vi "VP_NanoPositioner_FPGA_ModTrans.vi"() -> ()   [LabVIEW 2015]
uses:
  FPGA states.ctl
  FPGA Commands.ctl
  RT VIs/Scan type.ctl
  Data Save Trigger.ctl
  Scan Geometry.ctl
  spiral radial direction.ctl
  spiral rotation direction.ctl
  Inner Scan axis.ctl
  Scan Type and Geometry.ctl
  Data Save Flag.ctl
  <vilib>/Platform/TimedLoop/XDataNode/timing_clust.ctl
  <vilib>/Platform/TimedLoop/XDataNode/nitl_modes.ctl
  <vilib>/Platform/TimedLoop/XDataNode/wakeup.ctl
  Trajectory FGV states.ctl
  Transfer_function_coeffs.ctl
  Transfer_function_actions.ctl
  <vilib>/rvi/Emulation/niFpgaGetClockAttributes.vi
  <vilib>/rvi/Emulation/niFpgaSctlEmulationGetInTimedLoop.vi
  <vilib>/rvi/Emulation/niFpgaEmulationReportErrorSimple.vi
  <vilib>/rvi/Emulation/niFpgaEmulationIsFPGAContextNoSignature.vi
  <vilib>/rvi/DataTransferAndStorage/Container/Common/niFpgaContainerGetUniqueNameForEmu.vi
  <vilib>/rvi/Memory/Memory_Emulation/niFpgaMemoryEmulationCacheClearOnFirstRun.vi
  <vilib>/rvi/Memory/Memory_Emulation/nirvimemoryEmulationManagerCache_MakeExclusive.vi
  <vilib>/rvi/Memory/Memory_Emulation/niFpgaMemoryEmulationValidateCache.vi
  <vilib>/rvi/Memory/Memory_Emulation/nirvimemoryEmulationManagerCache_InsertValue.vi
  <vilib>/Utility/error.llb/Clear Errors.vi
  <vilib>/rvi/Memory/Memory_Emulation/nirvimemoryEmulationManagerCache_ReleaseExclusive.vi
  <vilib>/rvi/Memory/Memory_Emulation/nirvimemoryEmulationManagerCache_GetValue.vi
  <vilib>/rvi/Memory/Memory_Emulation/nirvimemoryEmulationManagerCache_SetValue.vi
  <vilib>/rvi/Emulation/niFpgaProcessEmulError.vi
  <vilib>/rvi/Emulation/niFpgaCriticalErrorInLSC.vi
  <vilib>/rvi/interface/RandomDataEmulation/niFpgaRandomDataHandleErrors.vi
  <vilib>/rvi/eio/common/nirviEmuTemplateMethod_errors.vi
  <vilib>/rvi/DataTransferAndStorage/Container/XNode/niFpgaContainer.xnode
  <vilib>/rvi/DataTransferAndStorage/Register/Emulation/niFpgaRegisterEmulation.vi
  <vilib>/rvi/interface/RandomDataEmulation/nirviRandomDataFpgaReadWriteTemplate.vi
  <vilib>/eio/EIONode/EIONode.xnode
  <vilib>/Platform/TimedLoop/XDataNode/XDataNode.xnode
  <vilib>/Platform/TimedLoop/XDataNode/XDNodeRunTimeDep.lvlib
panel:
  in  "Data Save Flag":T1=enum."Save Data"
  out "Position Number":u32
  out "Scan Type and Geometry":T2
  out "Outer Loop iterations":i32
  out "Counter Loop iterations":i32
  in  "Y Reference DC Offset (nm)":fxp<+/-,16,16>
  in  "Y Reference Amplitude (nm)":fxp<+/-,40,17>
  in  "X Reference DC Offset (nm)":fxp<+/-,16,16>
  in  "X Reference Amplitude (nm)":fxp<+/-,40,17>
  out "Controller loop iterations":i32
  out "Trajectory Complete":bool
  in  "Inner Scan axis":T3
  in  "Spiral Rotation Direction":T4
  in  "Radial direction":T5=enum."Inward"
  in  "Det Frequency":fxp<+,32,0>=0.9999999997671694
  in  "Traj Frequency":fxp<+,32,0>=0.9999999997671694
  in  "Max radius":fxp<+/-,32,16>
  in  "Spiral Step Size":fxp<+/-,32,16>
  in  "Y Step Size":fxp<+/-,24,16>
  in  "X Step Size":fxp<+/-,24,16>
  in  "Scan Geometry":T6
  out "Z Reference Loop iterations":i32
  out "XY Reference Loop iterations":i32
  in  "Data Save Trigger Source":T7
  out "FIFO loop iterations":i32
  out "Trigger Generation Loop iterations":i32
  out "Module output loop iterations":i32
  out "Plant output loop iterations":i32
  in  "Scan type":T8
  out "Interferometer Loop Error":errorcluster
  out "Wait error":errorcluster
  out "Shutdown error":errorcluster
  out "FPGA error monitor":errorcluster
  out "Run Loop error":errorcluster
  in  "Wait timer (ms)":u16=50 caption="Count(mSec)"
  in  "New FPGA command":bool
  in  "FPGA command":T9
  out "FPGA state":T10
  out "End Run Error":errorcluster
  in  "Y End (nm)":fxp<+/-,16,16>
  in  "Y Start (nm)":fxp<+/-,16,16>
  in  "X End (nm)":fxp<+/-,16,16>
  in  "X Start (nm)":fxp<+/-,16,16>
  in  "DT Reset":bool
  in  "DT Duty Cycle (periods)":fxp<+,32,0>=0.5 caption="DT duty cycle (periods)"
  in  "DT Reference DC Offset (V)":fxp<+/-,16,16>
  in  "DT Reference Amplitude (V)":fxp<+/-,40,17>
  in  "DT Phase Offset (periods)":fxp<+,32,0>
  out "Measured Z Reference Loop Period (ticks)":u32
  in  "Z Reference Loop Period (us)":u32 caption="Z Reference Time Period (uSec)"
  in  "Z Reference DC Offset (nm)":fxp<+/-,16,16>
  in  "Z Reference Amplitude (nm)":fxp<+/-,40,17>
  in  "Detector Trigger Lower Limit (V)":fxp<+/-,20,5>=-5.0
  out "Detector Trigger In Range?":bool
  in  "Detector Trigger Upper Limit (V)":fxp<+/-,20,5>=5.0
  out "Measured Trigger Generation Loop Period (Ticks)":u32
  in  "Trigger Generation Time Period (uSec)":u32
  in  "Z-Stage Scaling Direction":fxp<+/-,3,3>=-1.0
  in  "Y-Stage Scaling Direction":fxp<+/-,3,3>=-1.0
  in  "Optics and or Sample Stage":T11(ring)
  in  "Sample Z Stage Resolution (nm)":fxp<+,33,3>=0.001000046730041504
  in  "Sample Y Stage Resolution (nm)":fxp<+,33,3>=0.001000046730041504
  in  "Sample X Stage Resolution (nm)":fxp<+,33,3>=0.001000046730041504
  out "Sample Z Stage Displacement raw (nm)":fxp<+/-,32,16> format="%.62g"
  out "Sample Y Stage Displacement raw (nm)":fxp<+/-,32,16> format="%.41g"
  out "Sample X Stage Displacement raw (nm)":fxp<+/-,32,16> format="%.62g"
  in  "Reset Sample Z":bool
  in  "Reset Sample Y":bool
  in  "Reset Sample X":bool
  out "Mod6/DIO3":bool
  out "Mod6/DIO2":bool
  out "Mod5/DIO3":bool
  out "Mod5/DIO2":bool
  out "Mod4/DIO3":bool
  out "Mod4/DIO2":bool
  in  "X-Stage Scaling Direction":fxp<+/-,3,3>=-1.0
  in  "Z-Stage nm to V Scaling":fxp<+/-,32,12>
  in  "Y-Stage nm to V Scaling":fxp<+/-,32,12>
  in  "X-Stage nm to V Scaling":fxp<+/-,32,12>
  out "Kxx Output, Kxx*ex (V)":fxp<+/-,58,25>
  out "Kyy Output, Kyy*ey (V)":fxp<+/-,58,25>
  out "Kzz Output, Kzz*ez (V)":fxp<+/-,58,25>
  in  "sos gain SF Controller xx1":fxp<+/-,42,9>
  in  "-a01(2) xx1":fxp<+/-,64,9>[](array[numeric])=[0.0, 0.0, 0.0, 0.0, 0.0, 0.0, 0.0, 0.0, 0.0, 0.0, 0.0, 0.0, 0.0, 0.0, 0.0, 0.0, 0.0, 0.0, 0.0, 0.0]
  in  "-a02(2) xx1":fxp<+/-,64,9>[](array[numeric])=[0.0, 0.0, 0.0, 0.0, 0.0, 0.0, 0.0, 0.0, 0.0, 0.0, 0.0, 0.0, 0.0, 0.0, 0.0, 0.0, 0.0, 0.0, 0.0, 0.0]
  in  "b01(2) xx1":fxp<+/-,64,9>[](array[numeric])=[0.0, 0.0, 0.0, 0.0, 0.0, 0.0, 0.0, 0.0, 0.0, 0.0, 0.0, 0.0, 0.0, 0.0, 0.0, 0.0, 0.0, 0.0, 0.0, 0.0]
  in  "b02(2) xx1":fxp<+/-,64,9>[](array[numeric])=[0.0, 0.0, 0.0, 0.0, 0.0, 0.0, 0.0, 0.0, 0.0, 0.0, 0.0, 0.0, 0.0, 0.0, 0.0, 0.0, 0.0, 0.0, 0.0, 0.0]
  in  "sos gain SF Controller yy1":fxp<+/-,42,9>
  in  "-a01(2) yy1":fxp<+/-,64,9>[](array[numeric])=[0.0, 0.0, 0.0, 0.0, 0.0, 0.0, 0.0, 0.0, 0.0, 0.0, 0.0, 0.0, 0.0, 0.0, 0.0, 0.0, 0.0, 0.0, 0.0, 0.0]
  in  "-a02(2) yy1":fxp<+/-,64,9>[](array[numeric])=[0.0, 0.0, 0.0, 0.0, 0.0, 0.0, 0.0, 0.0, 0.0, 0.0, 0.0, 0.0, 0.0, 0.0, 0.0, 0.0, 0.0, 0.0, 0.0, 0.0]
  in  "b01(2) yy1":fxp<+/-,64,9>[](array[numeric])=[0.0, 0.0, 0.0, 0.0, 0.0, 0.0, 0.0, 0.0, 0.0, 0.0, 0.0, 0.0, 0.0, 0.0, 0.0, 0.0, 0.0, 0.0, 0.0, 0.0]
  in  "b02(2) yy1":fxp<+/-,64,9>[](array[numeric])=[0.0, 0.0, 0.0, 0.0, 0.0, 0.0, 0.0, 0.0, 0.0, 0.0, 0.0, 0.0, 0.0, 0.0, 0.0, 0.0, 0.0, 0.0, 0.0, 0.0]
  in  "sos gain SF Controller zz1":fxp<+/-,42,9>
  in  "-a01(2) zz1":fxp<+/-,64,9>[](array[numeric])=[0.0, 0.0, 0.0, 0.0, 0.0, 0.0, 0.0, 0.0, 0.0, 0.0, 0.0, 0.0, 0.0, 0.0, 0.0, 0.0, 0.0, 0.0, 0.0, 0.0]
  in  "-a02(2) zz1":fxp<+/-,64,9>[](array[numeric])=[0.0, 0.0, 0.0, 0.0, 0.0, 0.0, 0.0, 0.0, 0.0, 0.0, 0.0, 0.0, 0.0, 0.0, 0.0, 0.0, 0.0, 0.0, 0.0, 0.0]
  in  "b01(2) zz1":fxp<+/-,64,9>[](array[numeric])=[0.0, 0.0, 0.0, 0.0, 0.0, 0.0, 0.0, 0.0, 0.0, 0.0, 0.0, 0.0, 0.0, 0.0, 0.0, 0.0, 0.0, 0.0, 0.0, 0.0]
  in  "b02(2) zz1":fxp<+/-,64,9>[](array[numeric])=[0.0, 0.0, 0.0, 0.0, 0.0, 0.0, 0.0, 0.0, 0.0, 0.0, 0.0, 0.0, 0.0, 0.0, 0.0, 0.0, 0.0, 0.0, 0.0, 0.0]
  in  "Scaling mV to V":fxp<+,33,10>=0.0009765625
  in  "System Loop Type":enum16{"Open Loop", "Closed Loop"}(ring)
  in  "Timeout FPGA FIFO1":i32=40000000
  out "FIFO Timed Out":bool
  out "Number of Data Strings":i32
  out "Optics Z Stage Displacement raw (nm)":fxp<+/-,32,16>
  in  "Optics Z Stage Resolution (nm)":fxp<+,33,3>=0.001000046730041504
  in  "Reset Optics Z":bool
  out "Mod6/DIO1":bool
  out "Mod6/DIO0":bool
  out "Optics Y Stage Displacement raw (nm)":fxp<+/-,32,16>
  in  "Optics Y Stage Resolution (nm)":fxp<+,33,3>=0.001000046730041504
  in  "Reset Optics Y":bool
  out "Mod5/DIO1":bool
  out "Mod5/DIO0":bool
  out "Z-Stage Input In Range?":bool
  out "Y-Stage Input In Range?":bool
  in  "Controller Output Lower Limit":fxp<+/-,20,5>=-5.0
  out "X-Stage Input In Range?":bool
  in  "Controller Output Upper Limit":fxp<+/-,20,5>=5.0
  out "Measured Counter Time Period (Ticks)":u32
  out "Measured Datalog Period (Ticks)":u32
  out "Measured Plant Output Loop Period (Ticks)":u32
  out "Measured Module Output Loop Period (Ticks)":u32
  out "Measured Controller Loop Period (Ticks)":u32
  out "Measured XY Reference Loop Period (ticks)":u32
  out "Optics X Stage Displacement raw (nm)":fxp<+/-,32,16>
  in  "Optics X Stage Resolution (nm)":fxp<+,33,3>=0.001000046730041504 format="%#_31g"
  in  "Plant Output Loop Period (uSec)":u32 caption="Plant Output Time Period (uSec)"
  in  "Reset Optics X":bool
  out "Mod4/DIO1":bool
  out "Mod4/DIO0":bool
  out "Start Run Error":errorcluster
  out "Stop Scan":bool
  in  "Module Output Loop Period (uSec)":u32 caption="Controller Output Time Period (uSec)"
  in  "Datalog Cases":T12(ring)
  in  "Controller Loop Period (uSec)":u32 caption="Controller Time Period (uSec)"
  in  "FIFO Loop Period (us)":u32 caption="Datalog Time Period (uSec)"
  in  "XY Reference Loop Period (us)":u32 caption="X Reference Time Period (uSec)"
  out "FIFO Timed Out?":bool
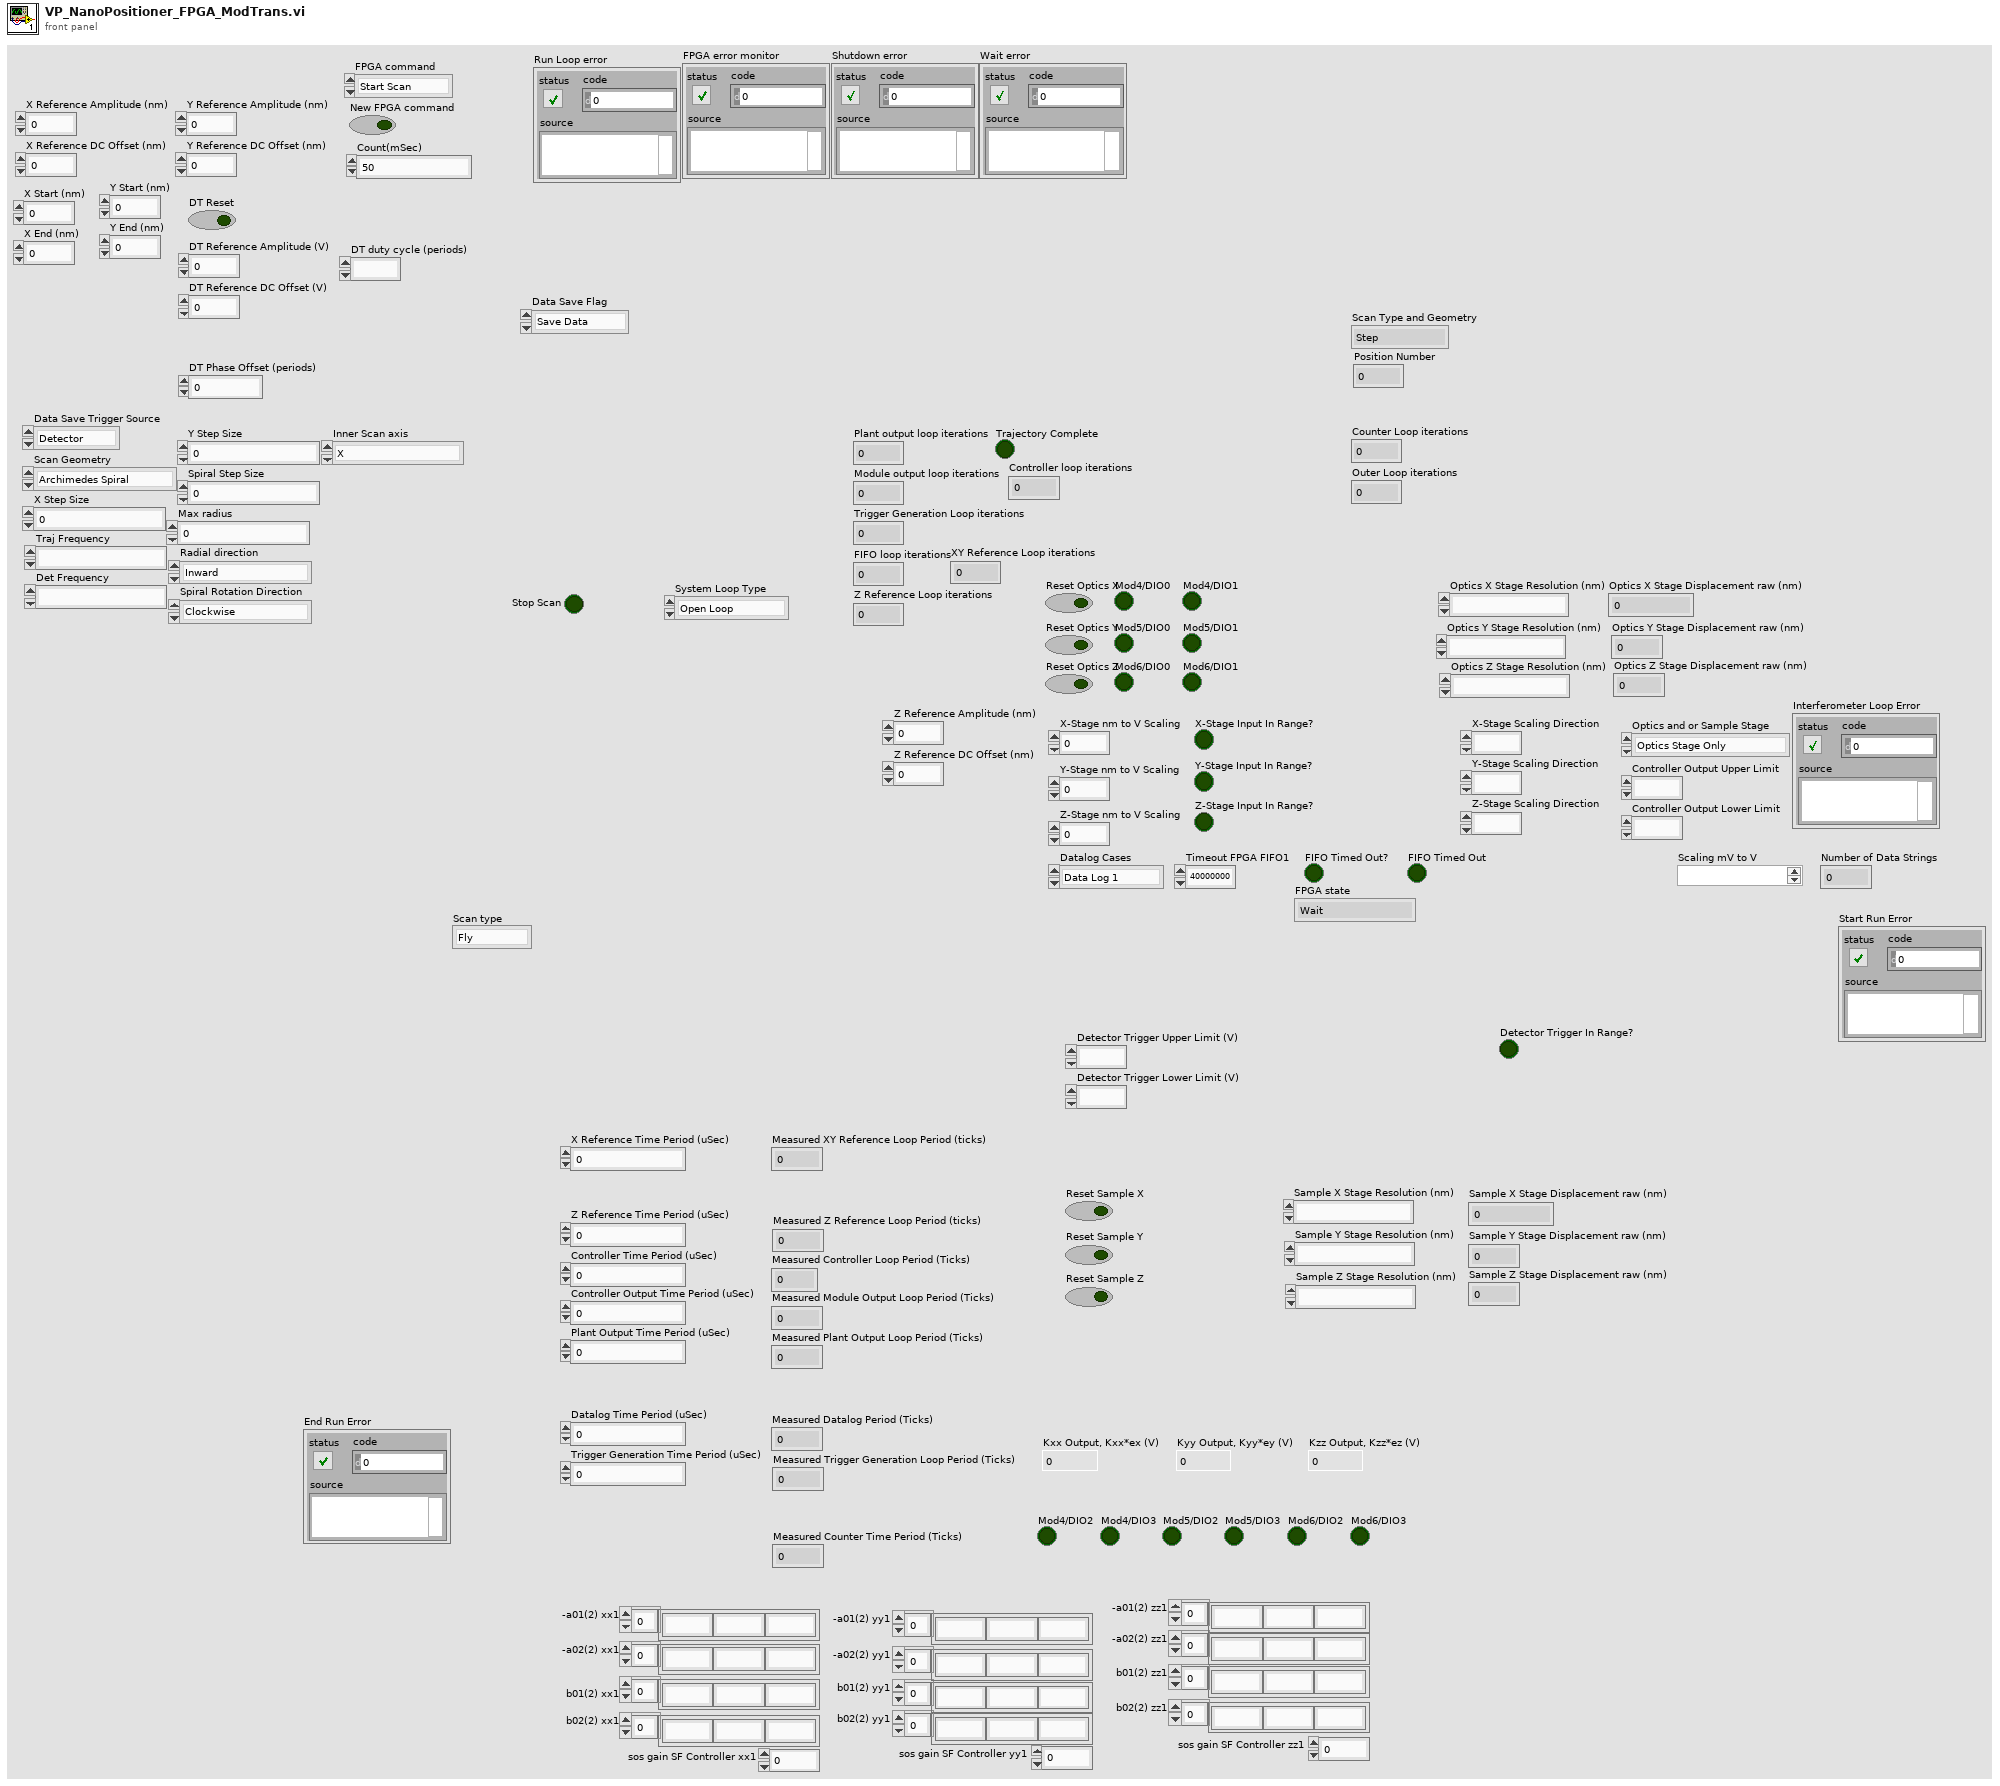
[diagram p1: front panel]
types:
  T1 = typedef "Data Save Flag.ctl" = enum16{"Skip Data", "Save Data"}
  T2 = typedef "Scan Type and Geometry.ctl" = enum16{"Step", "Fly Arch Spiral", "Fly Snake", "Fly Grid Spiral"}
  T3 = typedef "Inner Scan axis.ctl" = enum16{"X", "Y"}
  T4 = typedef "spiral rotation direction.ctl" = enum16{"Clockwise", "Anti-clockwise"}
  T5 = typedef "spiral radial direction.ctl" = enum16{"Outward", "Inward"}
  T6 = typedef "Scan Geometry.ctl" = enum16{"Archimedes Spiral", "Grid Spiral", "Snake"}
  T7 = typedef "Data Save Trigger.ctl" = enum16{"Detector", "Trajectory"}
  T8 = typedef "Scan type.ctl" = enum16{"Fly", "Step"}
  T9 = typedef "FPGA Commands.ctl" = enum16{"Start Scan", "Shutdown"}
  T10 = typedef "FPGA states.ctl" = enum16{"Wait", "Start Run", "Run", "End Run", "Shutdown"}
  T11 = enum16{"Optics Stage Only", "Optics and Sample Stage"}
  T12 = enum16{"Data Log 1", "Data Log 2", "Data Log 3", "Data Log 4", "Data Log 5", "Data Log 6", "Data Log 7", "Data Log 8", "Data Log 9", "Data Log 10", "Data Log 11", "Data Log 12", "Data Log 13", "Data Log 14", "Data Log 15", "Data Log 16"}
  T13 = typedef "Transfer_function_actions.ctl" = enum16{"Initialize", "Calculate"}
  T14 = typedef "Trajectory FGV states.ctl" = enum16{"Initialize", "Increment"}
  T15 = typedef "XDNodeRunTimeDep.lvlib/timing_clust.ctl" = cluster{"Expected End [f-1]":u64, "Actual End [f-1]":u64, "Finished Late? [f-1]":bool, "Expected End [i-1]":u64, "Actual End [i-1]":u64, "Finished Late? [i-1]":bool, "Expected Start [i]":u64, "Actual Start [i]":u64, "Expected Start [f]":u64, "Actual Start [f]":u64, "Source Name":string, "Structure Name":string, "Period":i64, "Deadline":i64, "Offset":i64, "Start":i64, "Priority":i32, "Timeout":i32, "Mode":T16, "Wakeup Reason":T17, "Error":errorcluster, "Source Type":string, "Secondary Source Type":string, "Global End Time":u64, "Global Start Time":u64, "Frame Duration":u64, "Iteration Duration":u64, "Assigned CPU":i32, "I/O Scan Engine Mode":u32}
  T16 = typedef "XDNodeRunTimeDep.lvlib/nitl_modes.ctl" = enum32{"No Change", "Process missed periods, maintain original phase", "Discard missed periods, maintain original phase", "Process missed periods, ignore original phase", "Discard missed periods, ignore original phase"}
  T17 = typedef "XDNodeRunTimeDep.lvlib/wakeup.ctl" = enum32{"Normal", "Aborted", "Asynchronous wakeup", "Timing source error", "Timed loop error", "Timeout"}
  T18 = typedef "Transfer_function_coeffs.ctl" = cluster{"sos gain SF Controller":fxp<+/-,42,9>, "-a01(2)":fxp<+/-,64,9>[], "-a02(2)":fxp<+/-,64,9>[], "b01(2)":fxp<+/-,64,9>[], "b02(2)":fxp<+/-,64,9>[]}
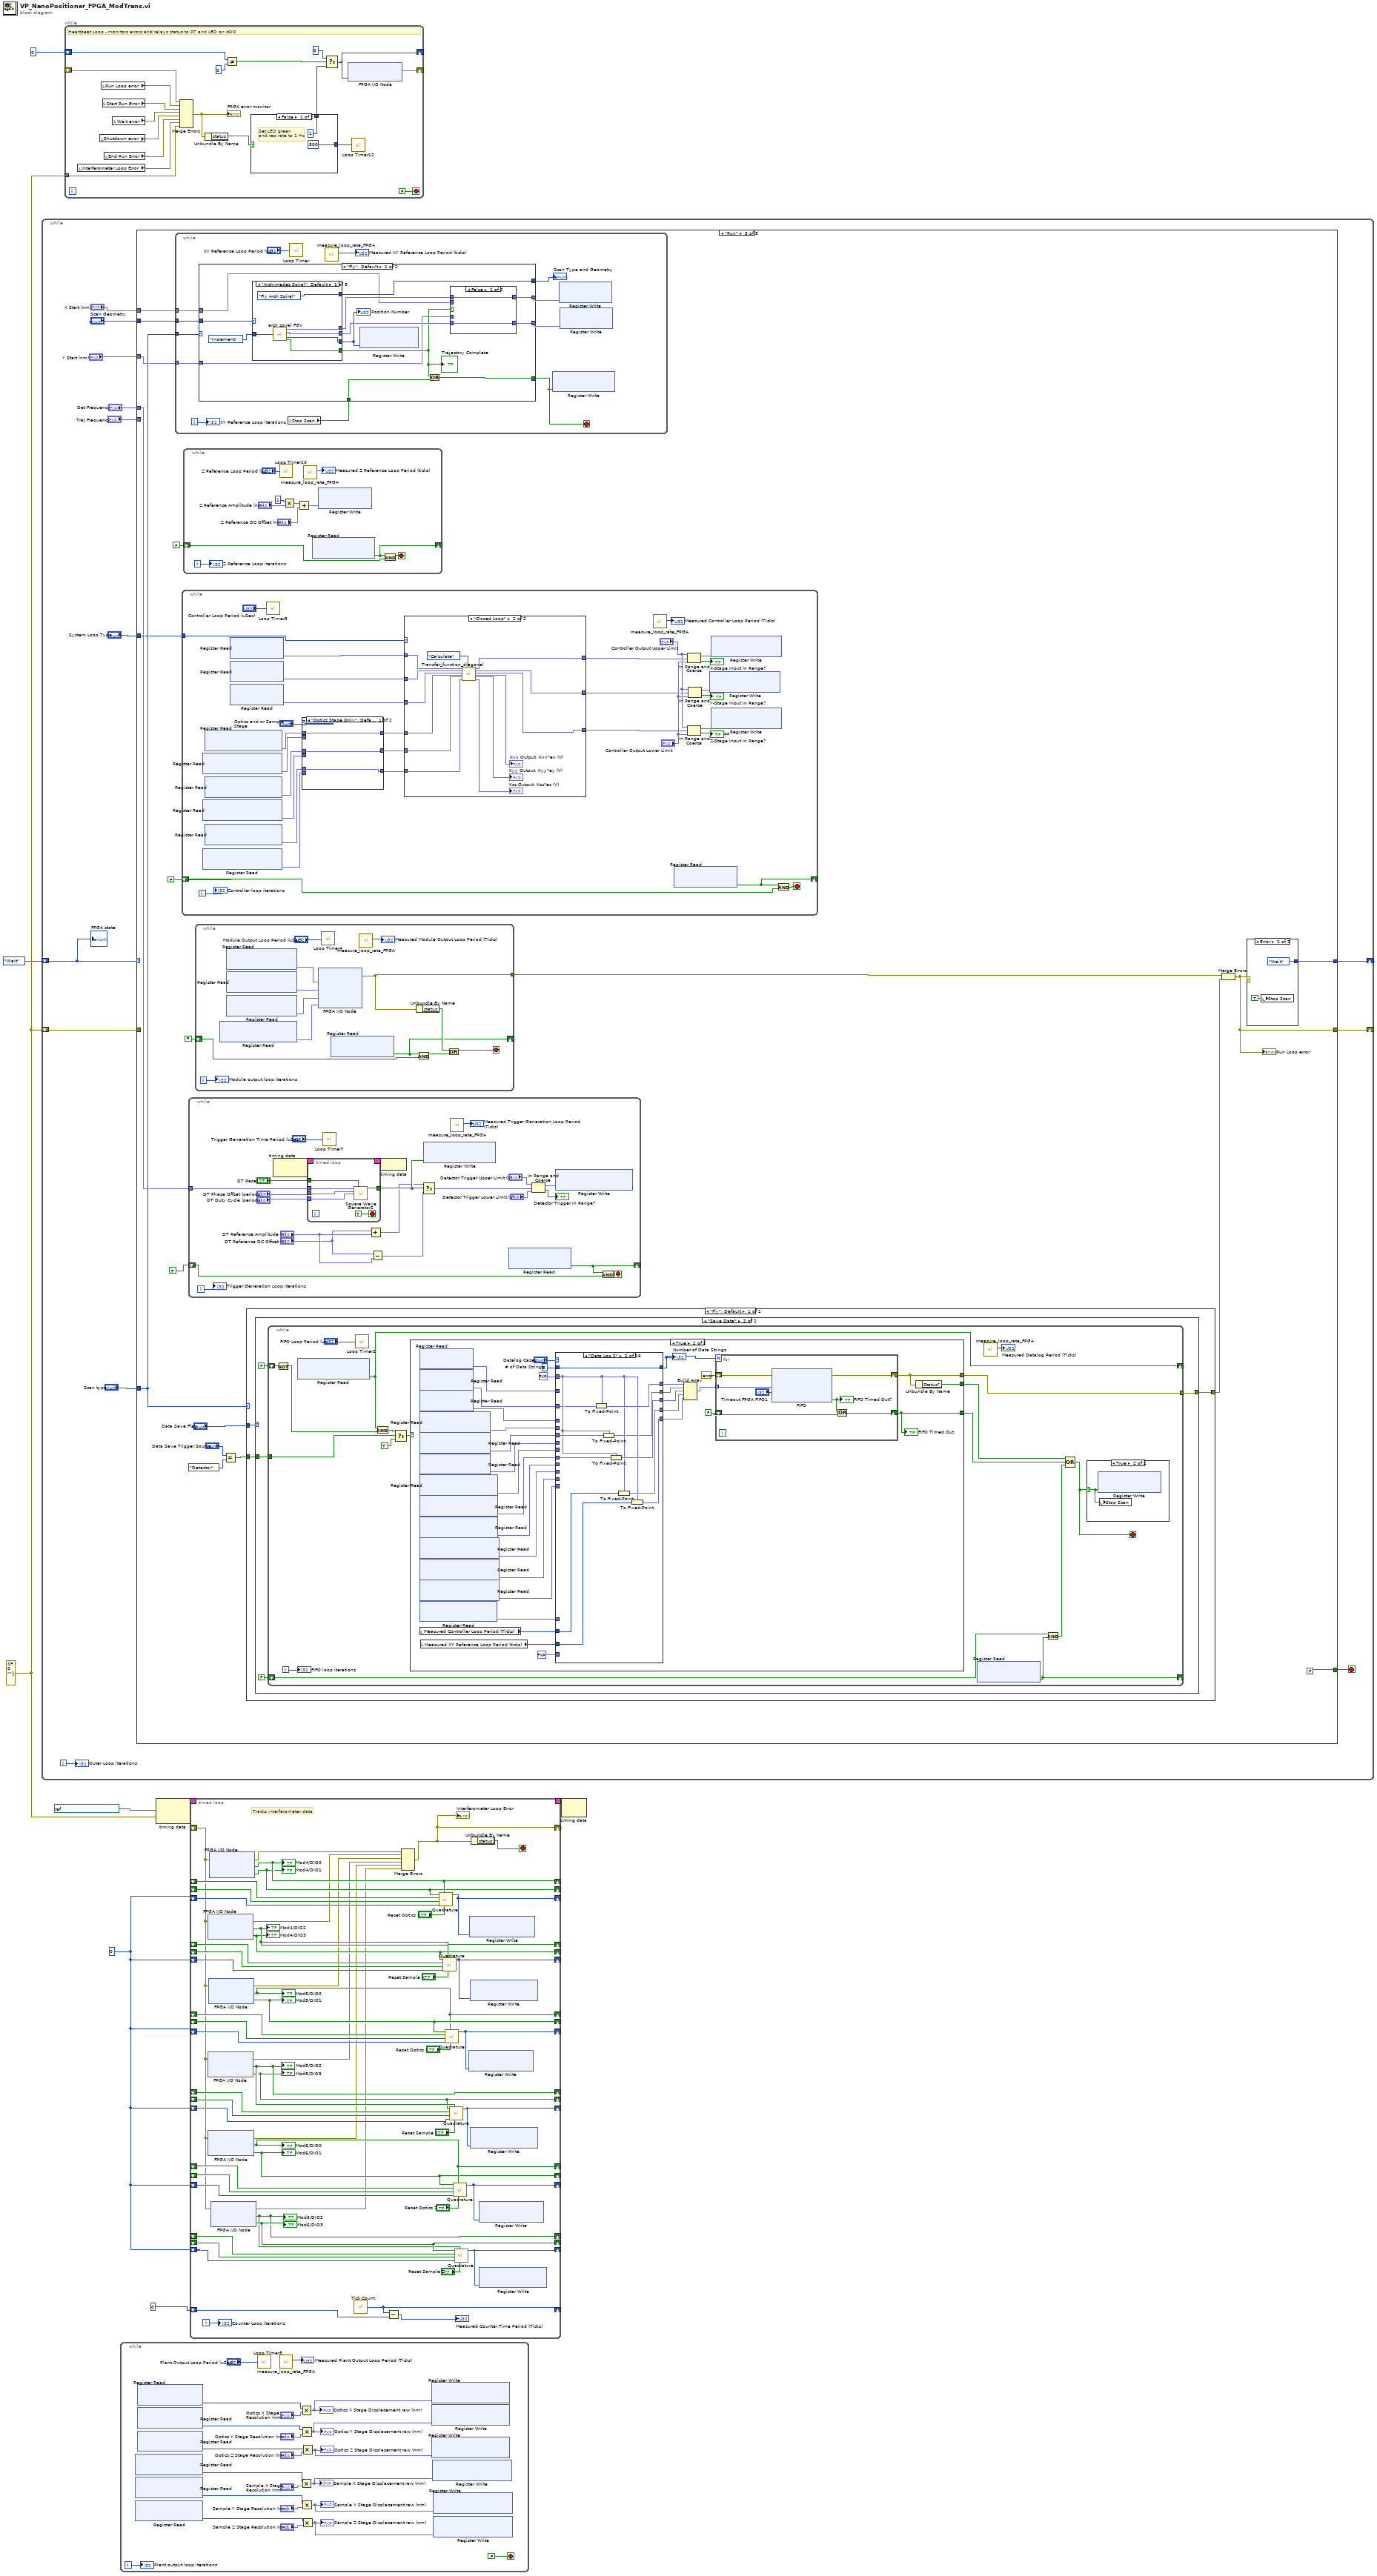
[diagram p0: block diagram]
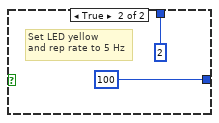
[diagram p2: hidden frame]
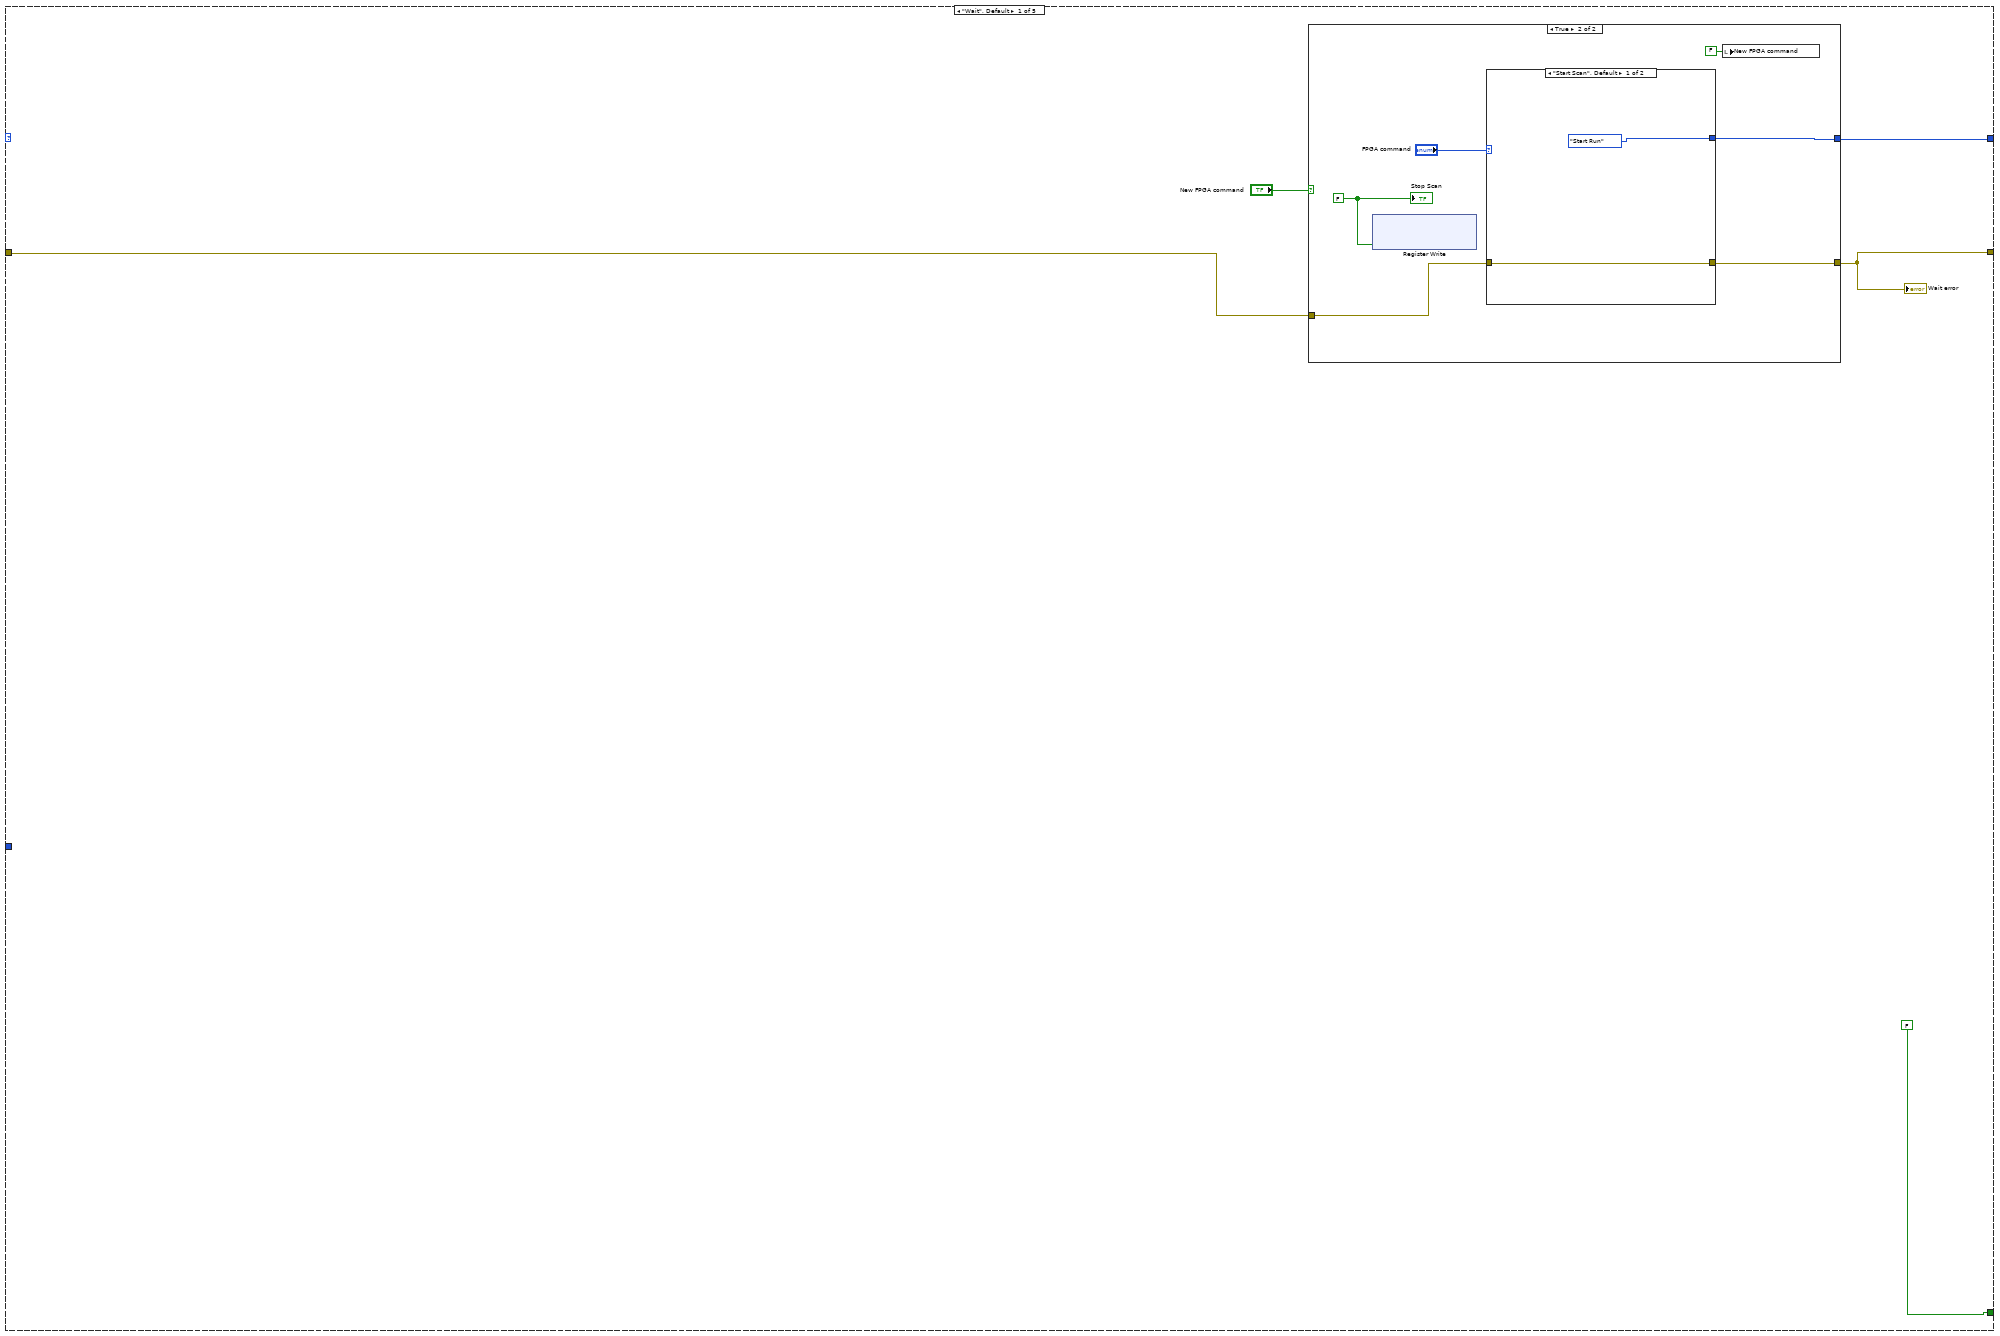
[diagram p3: hidden frame]
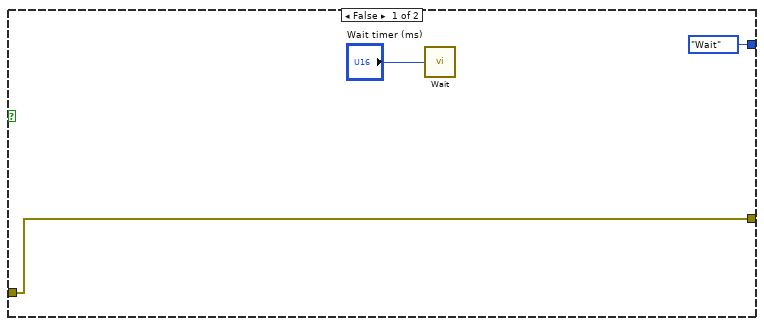
[diagram p4: hidden frame]
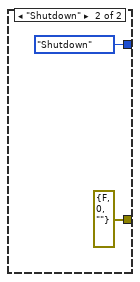
[diagram p5: hidden frame]
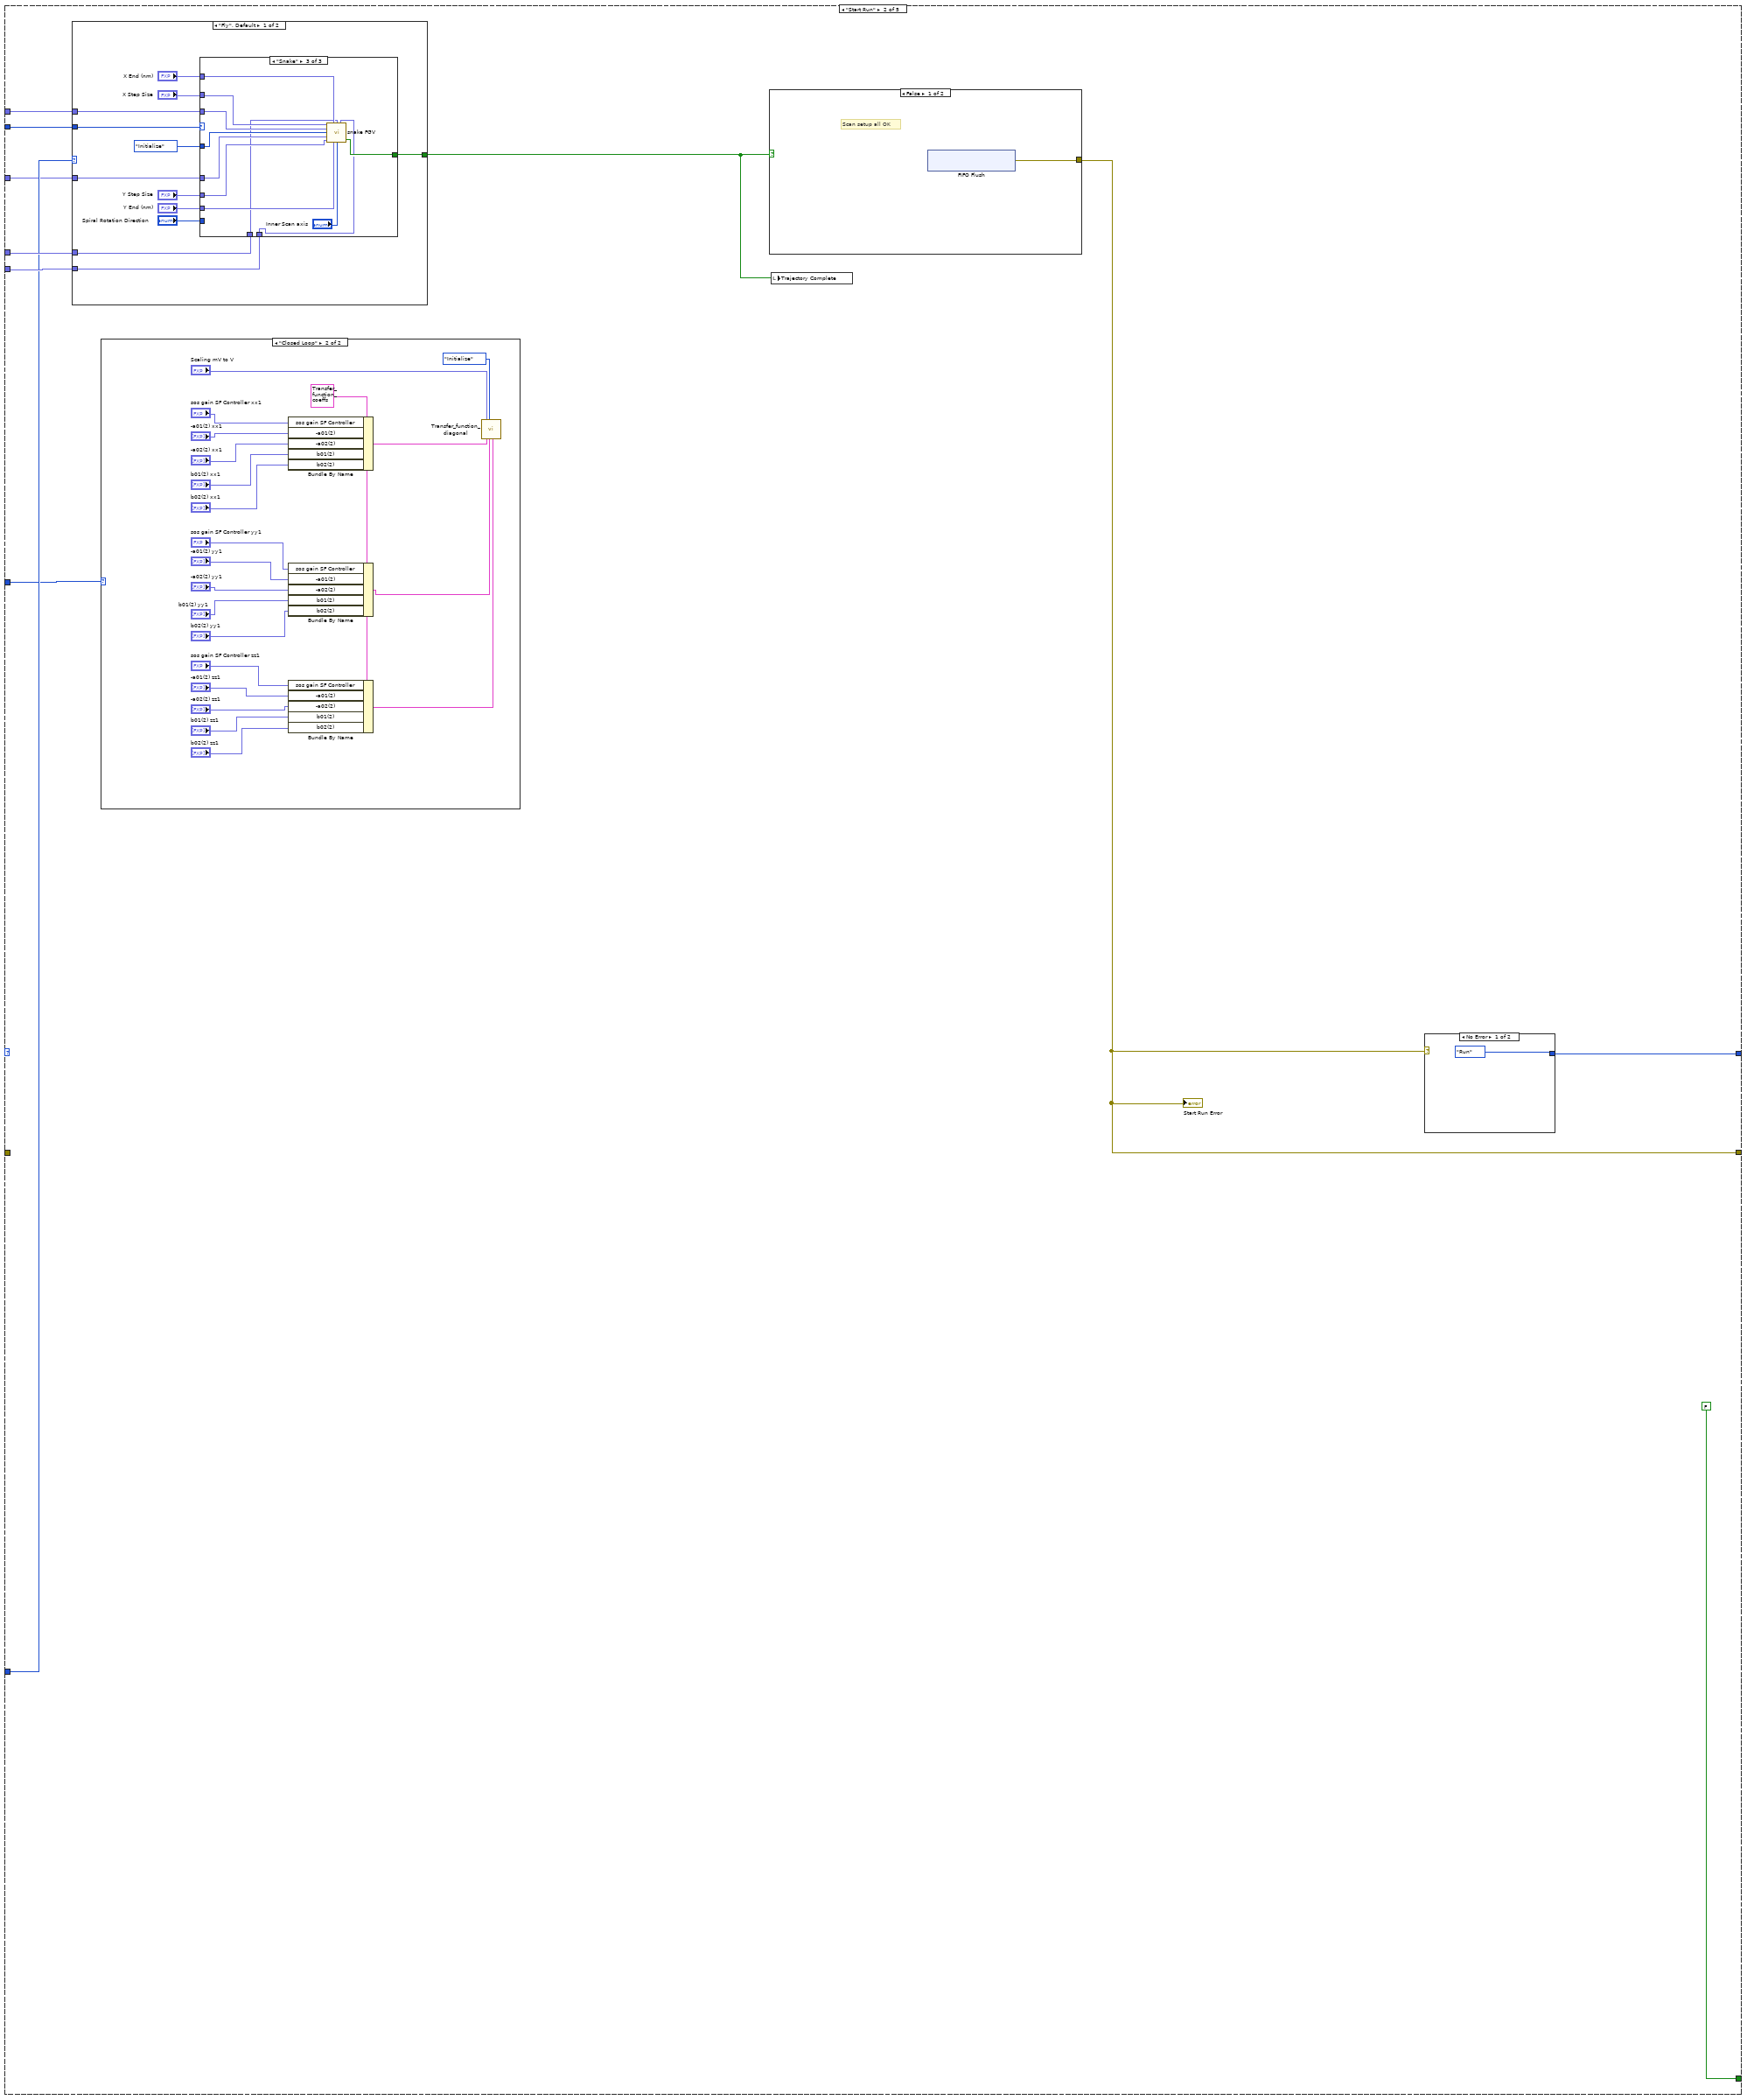
[diagram p6: hidden frame]
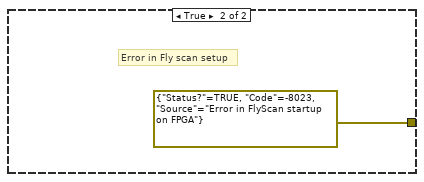
[diagram p8: hidden frame]
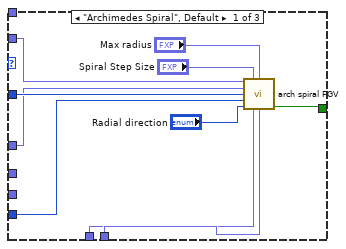
[diagram p9: hidden frame]
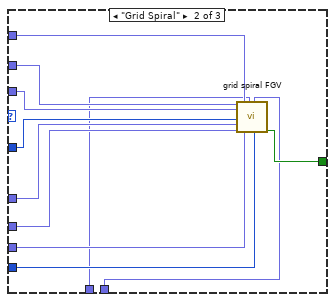
[diagram p10: hidden frame]
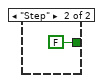
[diagram p11: hidden frame]
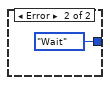
[diagram p12: hidden frame]
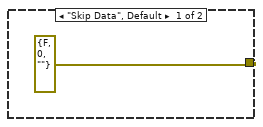
[diagram p13: hidden frame]
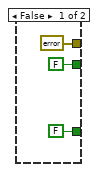
[diagram p14: hidden frame]
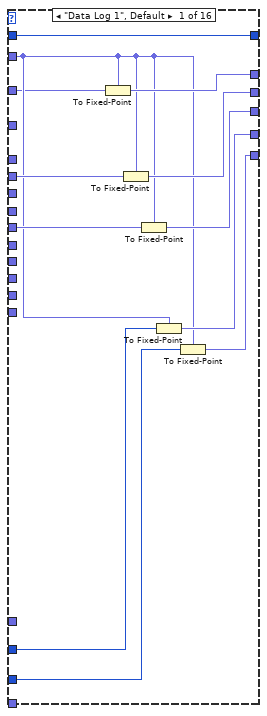
[diagram p15: hidden frame]
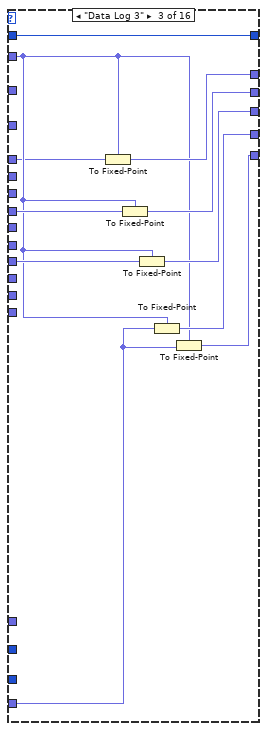
[diagram p16: hidden frame]
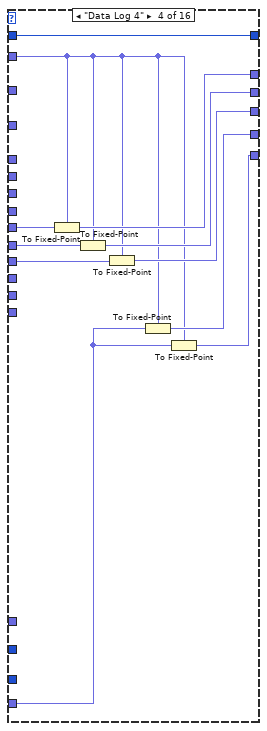
[diagram p17: hidden frame]
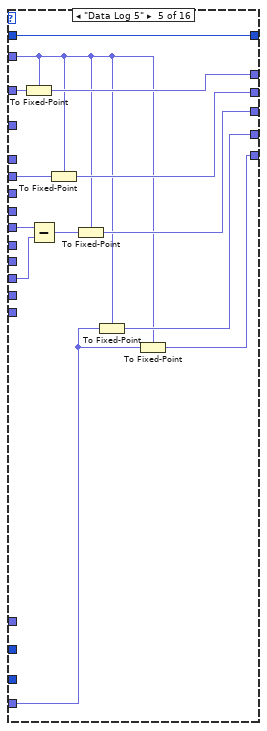
[diagram p18: hidden frame]
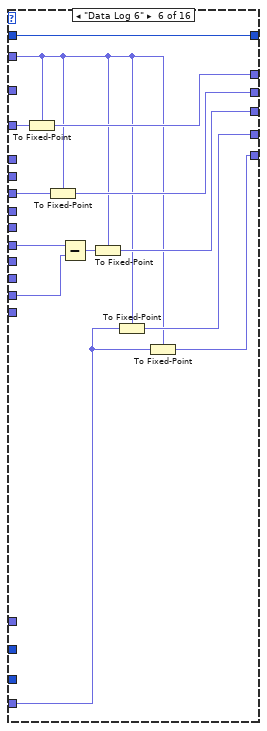
[diagram p19: hidden frame]
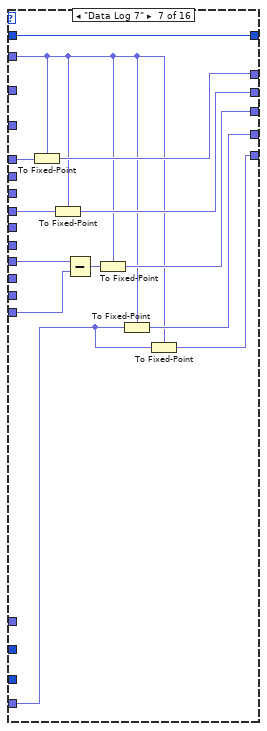
[diagram p20: hidden frame]
diagram:
  w4 = 0 ("Tick Count(Ticks)")
  w1 = errorcluster {"status"=FALSE, "code"=0, "source"=""} ("error IO")
  n1 = while {
    shift-right: [w14] -> _
    shift-left: FPGA_states."Wait" -> [w21]
    shift-right: [w19] -> _
    shift-left: w1 -> [w10]
    i -> [w13]
    stop <- w20 stop-if-true
    n2 = case shown="\"Run\"" w21 {
      tunnel: [w26 w44 w137 w584 w591] -> w19
      tunnel: [FALSE FALSE FALSE FALSE TRUE] -> w20
      tunnel: [w23 w45 w138 FPGA_states."Wait" FPGA_states."Shutdown"] -> w14
      tunnel: w10 -> [w24 _ _ w585 w592]
      tunnel: "Scan Geometry" -> [_ w49 w134 _ _]
      tunnel: "Traj Frequency" -> [_ w48 _ _ _]
      tunnel: "Det Frequency" -> [_ w47 w129 _ _]
      tunnel: "Scan type" -> [_ w46 w130 _ _]
      tunnel: "X Start (nm)" -> [_ w42 w124 _ _]
      tunnel: "Y Start (nm)" -> [_ w41 w125 _ _]
      tunnel: "System Loop Type" -> [_ w40 w121 _ _]
      frame "Wait", Default {
        n3 = case shown="True" "New FPGA command" {
          tunnel: [FPGA_states."Wait" w35] -> w23
          tunnel: w24 -> [w29 w34]
          tunnel: [w29 w33] -> w26
          frame False {
            n4 = call "Wait"("Count(mSec)"="Wait timer (ms)") -> ()  [unwired: 1 out]
          }
          frame True {
            w30 = FALSE ("stop case")
            n5 = xnode ("Register Write")("Data"=w30) -> ()  [unwired: 1 in, 1 out]
            n6 = case shown="\"Start Scan\", Default" "FPGA command" {
              tunnel: [FPGA_states."Start Run" FPGA_states."Shutdown"] -> w35
              tunnel: w34 -> [w36 _]
              tunnel: [w36 errorcluster {"status"=FALSE, "code"=0, "source"=""} ("error IO")] -> w33
              frame "Start Scan", Default {
              }
              frame "Shutdown" {
              }
            }
            n7 = local write "New FPGA command"(FALSE ("New FPGA command")) -> ()
            "Stop Scan" <- w30
          }
        }
        "Wait error" <- w26
      }
      frame "Start Run" {
        n8 = case shown="\"Fly\", Default" w46 {
          tunnel: w49 -> [w84 _]
          tunnel: w48 -> [w83 _]
          tunnel: w47 -> [w82 _]
          tunnel: [w76 FALSE ("Trajectory Complete")] -> w43
          tunnel: w42 -> [w75 _]
          tunnel: w41 -> [w74 _]
          frame "Fly", Default {
            n9 = case shown="\"Snake\"" w84 {
              tunnel: Trajectory_FGV_states."Initialize" ("Action") -> [w95 w106 w117]
              tunnel: [w94 w105 w116] -> w76
              tunnel: w75 -> [w93 w104 w115]
              tunnel: "X Step Size" -> [_ w103 w114]
              tunnel: "X End (nm)" -> [_ w102 w113]
              tunnel: w74 -> [w92 w101 w112]
              tunnel: "Y Step Size" -> [_ w100 w111]
              tunnel: "Y End (nm)" -> [_ w99 w110]
              tunnel: w83 -> [w89 w96 w108]
              tunnel: w82 -> [w88 w97 w109]
              tunnel: "Spiral Rotation Direction" -> [w86 w98 _]
              frame "Archimedes Spiral", Default {
                n10 = call "arch spiral FGV.vi"("X Start"=w93, "Spiral Step Size"="Spiral Step Size", "Max radius"="Max radius", "Y Start"=w92, "Action"=w95, "Spiral Rotation Direction"=w86, "Radial direction"="Radial direction", "Det Frequency"=w88, "Traj Frequency"=w89) -> ("Trajectory Complete"=w94:bool)  [unwired: 3 in, 3 out]
              }
              frame "Grid Spiral" {
                n11 = call "grid spiral FGV.vi"("X Step Size"=w103, "X Start"=w104, "Action"=w106, "Y Start"=w101, "Y Step Size"=w100, "X End"=w102, "Y End"=w99, "Det Frequency"=w97, "Traj Frequency"=w96, "Spiral Rotation Direction"=w98) -> ("Trajectory Complete"=w105:bool)  [unwired: 2 in, 7 out]
              }
              frame "Snake" {
                n12 = call "snake FGV.vi"("X Step Size"=w114, "X End"=w113, "Det Frequency"=w109, "Traj Frequency"=w108, "X Start"=w115, "Action"=w117, "Y Start"=w112, "Y Step Size"=w111, "Y End"=w110, "Inner Scan axis"="Inner Scan axis") -> ("Trajectory Complete"=w116:bool)  [unwired: 2 in, 3 out]
              }
            }
          }
          frame "Step" {
          }
        }
        n13 = case shown="\"Closed Loop\"" w40 {
          frame "Open Loop", Default {
          }
          frame "Closed Loop" {
            w71 = T18 {"sos gain SF Controller"=0.0, "-a01(2)"=[0.0, 0.0, 0.0, 0.0, 0.0, 0.0, 0.0, 0.0, 0.0, 0.0, 0.0, 0.0, 0.0, 0.0, 0.0, 0.0, 0.0, 0.0, 0.0, 0.0], "-a02(2)"=[0.0, 0.0, 0.0, 0.0, 0.0, 0.0, 0.0, 0.0, 0.0, 0.0, 0.0, 0.0, 0.0, 0.0, 0.0, 0.0, 0.0, 0.0, 0.0, 0.0], "b01(2)"=[0.0, 0.0, 0.0, 0.0, 0.0, 0.0, 0.0, 0.0, 0.0, 0.0, 0.0, 0.0, 0.0, 0.0, 0.0, 0.0, 0.0, 0.0, 0.0, 0.0], "b02(2)"=[0.0, 0.0, 0.0, 0.0, 0.0, 0.0, 0.0, 0.0, 0.0, 0.0, 0.0, 0.0, 0.0, 0.0, 0.0, 0.0, 0.0, 0.0, 0.0, 0.0]} ("Transfer Function coeffs")
            n14 = Bundle By Name(cluster=w71, "sos gain SF Controller"="sos gain SF Controller xx1", "-a01(2)"="-a01(2) xx1", "-a02(2)"="-a02(2) xx1", "b01(2)"="b01(2) xx1", "b02(2)"="b02(2) xx1") -> (w53:T18)
            n15 = Bundle By Name(cluster=w71, "sos gain SF Controller"="sos gain SF Controller yy1", "-a01(2)"="-a01(2) yy1", "-a02(2)"="-a02(2) yy1", "b01(2)"="b01(2) yy1", "b02(2)"="b02(2) yy1") -> (w52:T18)
            n16 = Bundle By Name(cluster=w71, "sos gain SF Controller"="sos gain SF Controller zz1", "-a01(2)"="-a01(2) zz1", "-a02(2)"="-a02(2) zz1", "b01(2)"="b01(2) zz1", "b02(2)"="b02(2) zz1") -> (w51:T18)
            n17 = call "Transfer_function_diagonal.vi"("Scaling mV to V"="Scaling mV to V", "xx1 Transfer Function"=w53, "Action"=Transfer_function_actions."Initialize", "yy1 Transfer Function"=w52, "zz1 Transfer Function"=w51) -> ()  [unwired: 9 in, 6 out]
          }
        }
        n18 = case shown="False" w43 {
          tunnel: [w72 errorcluster {"Status?"=TRUE, "Code"=-8023, "Source"="Error in FlyScan startup on FPGA"} ("error out")] -> w44
          frame False {
            # "Scan setup all OK"
            n19 = xnode ("FIFO Flush")() -> ("error out"=w72:errorcluster)  [unwired: 2 in, 1 out]
          }
          frame True {
            # "Error in Fly scan setup"
          }
        }
        "Start Run Error" <- w44
        n20 = local write "Trajectory Complete"(w43) -> ()
        n21 = case shown="No Error" w44 {
          tunnel: [FPGA_states."Run" FPGA_states."Wait"] -> w45
          frame No Error {
          }
          frame Error {
          }
        }
      }
      frame "Run" {
        n22 = while {
          tunnel: w134 -> [w537]
          tunnel: w130 -> [w532]
          tunnel: w125 -> [w530]
          tunnel: w124 -> [w529]
          i -> [w538]
          stop <- w533 stop-if-true
          n23 = local read "Stop Scan"() -> (w534:bool)
          n24 = case shown="\"Fly\", Default" w532 {
            tunnel: w537 -> [w553 _]
            tunnel: [w546 w580] -> w536
            tunnel: [w544 w577] -> w535
            tunnel: w534 -> [w550 w583]
            tunnel: [w549 w583] -> w533
            tunnel: [w548 Scan_Type_and_Geometry."Step"] -> w531
            tunnel: w530 -> [w542 _]
            tunnel: w529 -> [w541 _]
            frame "Fly", Default {
              n25 = case shown="\"Archimedes Spiral\", Default" w553 {
                tunnel: Trajectory_FGV_states."Increment" ("Action") -> [w563 w569 w575]
                tunnel: [w562 w568 w574] -> w543
                tunnel: [w561 w567 w573] -> w547
                tunnel: [w560 w566 w572] -> w545
                tunnel: [w559 w565 w571] -> w551
                tunnel: [Scan_Type_and_Geometry."Fly Arch Spiral" Scan_Type_and_Geometry."Fly Grid Spiral" Scan_Type_and_Geometry."Fly Snake"] -> w548
                frame "Archimedes Spiral", Default {
                  n26 = call "arch spiral FGV.vi"("Action"=w563) -> ("X position"=w561:fxp<+/-,32,16>, "Y position"=w560:fxp<+/-,32,16>, "Number of positions"=w559:u32, "Trajectory Complete"=w562:bool)  [unwired: 11 in]
                }
                frame "Grid Spiral" {
                  n27 = call "grid spiral FGV.vi"("Action"=w569) -> ("X position"=w567:fxp<+/-,32,16>, "Y position"=w566:fxp<+/-,32,16>, "Number of positions"=w565:u32, "Trajectory Complete"=w568:bool)  [unwired: 11 in, 4 out]
                }
                frame "Snake" {
                  n28 = call "snake FGV.vi"("Action"=w575) -> ("X position"=w573:fxp<+/-,32,16>, "Y position"=w572:fxp<+/-,32,16>, "Number of positions"=w571:u32, "Trajectory Complete"=w574:bool)  [unwired: 11 in]
                }
              }
              "Trajectory Complete" <- w543
              "Position Number" <- w551
              n29 = xnode ("Register Write")("Data"=w551) -> ()  [unwired: 1 in, 1 out]
              n30 = Or(x=w543, y=w550) -> (x .or. y?=w549:bool)
              n31 = case shown="False" w543 {
                tunnel: w547 -> [w555 _]
                tunnel: [w555 w556] -> w546
                tunnel: w545 -> [w554 _]
                tunnel: [w554 w557] -> w544
                tunnel: w542 -> [_ w557]
                tunnel: w541 -> [_ w556]
                frame False {
                }
                frame True {
                }
              }
            }
            frame "Step" {
              n32 = Add(x="X Reference Amplitude (nm)", y="X Reference DC Offset (nm)") -> (x+y=w580:fxp<+/-,32,16>)
              n33 = Add(x="Y Reference Amplitude (nm)", y="Y Reference DC Offset (nm)") -> (x+y=w577:fxp<+/-,32,16>)
            }
          }
          "Scan Type and Geometry" <- w531
          n34 = call "Loop Timer"("Count(uSec)"="XY Reference Loop Period (us)") -> ()  [unwired: 1 out]
          n35 = call "measure_loop_rate_FPGA.vi"() -> ("Loop Rate (Ticks)"=→"Measured XY Reference Loop Period (ticks)":u32)  [unwired: 11 in]
          n36 = xnode ("Register Write")("Data"=w533) -> ()  [unwired: 1 in, 1 out]
          n37 = xnode ("Register Write")("Data"=w536) -> ()  [unwired: 1 in, 1 out]
          n38 = xnode ("Register Write")("Data"=w535) -> ()  [unwired: 1 in, 1 out]
          "XY Reference Loop iterations" <- w538
        }
        n39 = while {
          shift-right: [w459] -> _
          shift-left: FALSE ("Data") -> [w460]
          tunnel: w121 -> [w458]
          i -> [w468]
          stop <- w461 stop-if-true
          n40 = xnode ("Register Read")() -> ("Data"=w473:fxp<+/-,32,16>)  [unwired: 1 in, 1 out]
          n41 = xnode ("Register Read")() -> ("Data"=w471:fxp<+/-,32,16>)  [unwired: 1 in, 1 out]
          n42 = xnode ("Register Read")() -> ("Data"=w469:fxp<+/-,32,16>)  [unwired: 1 in, 1 out]
          n43 = xnode ("Register Read")() -> ("Data"=w474:fxp<+/-,32,16>)  [unwired: 1 in, 1 out]
          n44 = xnode ("Register Read")() -> ("Data"=w472:fxp<+/-,32,16>)  [unwired: 1 in, 1 out]
          n45 = xnode ("Register Read")() -> ("Data"=w470:fxp<+/-,32,16>)  [unwired: 1 in, 1 out]
          n46 = xnode ("Register Read")() -> ("Data"=w477:fxp<+/-,32,16>)  [unwired: 1 in, 1 out]
          n47 = xnode ("Register Read")() -> ("Data"=w476:fxp<+/-,32,16>)  [unwired: 1 in, 1 out]
          n48 = xnode ("Register Read")() -> ("Data"=w475:fxp<+/-,32,16>)  [unwired: 1 in, 1 out]
          n49 = call "Loop Timer3"("Count(uSec)"="Controller Loop Period (uSec)") -> ()  [unwired: 1 out]
          n50 = case shown="\"Optics Stage Only\", Default" "Optics and or Sample Stage" {
            tunnel: w473 -> [_ w500]
            tunnel: w474 -> [w491 w499]
            tunnel: [w491 w498] -> w482
            tunnel: w471 -> [_ w497]
            tunnel: w472 -> [w490 w496]
            tunnel: [w490 w495] -> w481
            tunnel: w469 -> [_ w494]
            tunnel: w470 -> [w489 w493]
            tunnel: [w489 w492] -> w480
            frame "Optics Stage Only", Default {
            }
            frame "Optics and Sample Stage" {
              n51 = Subtract(x=w499, y=w500) -> (x-y=w498:fxp<+/-,33,17>)
              n52 = Subtract(x=w496, y=w497) -> (x-y=w495:fxp<+/-,33,17>)
              n53 = Subtract(x=w493, y=w494) -> (x-y=w492:fxp<+/-,33,17>)
            }
          }
          n54 = case shown="\"Closed Loop\"" w458 {
            tunnel: w482 -> [_ w518]
            tunnel: w477 -> [w506 w527]
            tunnel: [w503 w525] -> w463
            tunnel: [w504 w526] -> w464
            tunnel: w481 -> [_ w517]
            tunnel: w476 -> [w501 w520]
            tunnel: w475 -> [w505 w519]
            tunnel: w480 -> [_ w516]
            tunnel: [w502 w524] -> w462
            frame "Open Loop", Default {
              n55 = Multiply(x="Y-Stage nm to V Scaling", y="Y-Stage Scaling Direction") -> (x*y=w510:fxp<+/-,35,15>)
              n56 = Multiply(x="X-Stage nm to V Scaling", y="X-Stage Scaling Direction") -> (x*y=w514:fxp<+/-,35,15>)
              n57 = Multiply(x="Z-Stage nm to V Scaling", y="Z-Stage Scaling Direction") -> (x*y=w509:fxp<+/-,35,15>)
              n58 = Multiply(x=w506, y=w514) -> (x*y=w504:fxp<+/-,32,16>)
              n59 = Multiply(x=w501, y=w510) -> (x*y=w503:fxp<+/-,32,16>)
              n60 = Multiply(x=w505, y=w509) -> (x*y=w502:fxp<+/-,32,16>)
            }
            frame "Closed Loop" {
              n61 = call "Transfer_function_diagonal.vi"("X reference"=w527, "Y reference"=w520, "Z reference"=w519, "X actual"=w518, "Y actual"=w517, "Z actual"=w516, "Action"=Transfer_function_actions."Calculate") -> ("X-stage voltage"=w526:fxp<+/-,32,16>, "Y-stage voltage"=w525:fxp<+/-,32,16>, "Z-stage voltage"=w524:fxp<+/-,32,16>, "Kxx Output, Kxx*ex (V)"=→"Kxx Output, Kxx*ex (V)":fxp<+/-,58,25>, "Kyy Output, Kyy*ey (V)"=→"Kyy Output, Kyy*ey (V)":fxp<+/-,58,25>, "Kzz Output, Kzz*ez (V)"=→"Kzz Output, Kzz*ez (V)":fxp<+/-,58,25>)  [unwired: 7 in]
            }
          }
          n62 = call "measure_loop_rate_FPGA.vi"() -> ("Loop Rate (Ticks)"=→"Measured Controller Loop Period (Ticks)":u32)  [unwired: 11 in]
          n63 = xnode ("Register Read")() -> ("Data"=w459:bool)  [unwired: 1 in, 1 out]
          n64 = In Range and Coerce(upper limit="Controller Output Upper Limit", x=w464, lower limit="Controller Output Lower Limit") -> (coerced(x)=w467:fxp<+/-,32,16>, In Range?=→"X-Stage Input In Range?":bool)
          n65 = In Range and Coerce(upper limit="Controller Output Upper Limit", x=w462, lower limit="Controller Output Lower Limit") -> (coerced(x)=w465:fxp<+/-,32,16>, In Range?=→"Z-Stage Input In Range?":bool)
          n66 = In Range and Coerce(upper limit="Controller Output Upper Limit", x=w463, lower limit="Controller Output Lower Limit") -> (coerced(x)=w466:fxp<+/-,32,16>, In Range?=→"Y-Stage Input In Range?":bool)
          n67 = xnode ("Register Write")("Data"=w466) -> ()  [unwired: 1 in, 1 out]
          n68 = xnode ("Register Write")("Data"=w467) -> ()  [unwired: 1 in, 1 out]
          n69 = xnode ("Register Write")("Data"=w465) -> ()  [unwired: 1 in, 1 out]
          n70 = And(x=w459, y=w460) -> (x .and. y?=w461:bool)
          "Controller loop iterations" <- w468
        }
        n71 = while {
          shift-right: [w403] -> _
          shift-left: FALSE ("Data") -> [w402]
          i -> [w405]
          stop <- w404 stop-if-true
          n72 = call "Loop Timer10"("Count(uSec)"="Z Reference Loop Period (us)") -> ()  [unwired: 1 out]
          n73 = Multiply(x=i16 1 ("y"), y="Z Reference Amplitude (nm)") -> (x*y=w407:fxp<+/-,56,33>)
          n74 = Add(x=w407, y="Z Reference DC Offset (nm)") -> (x+y=w406:fxp<+/-,32,16>)
          n75 = call "measure_loop_rate_FPGA.vi"() -> ("Loop Rate (Ticks)"=→"Measured Z Reference Loop Period (ticks)":u32)  [unwired: 11 in]
          n76 = xnode ("Register Read")() -> ("Data"=w403:bool)  [unwired: 1 in, 1 out]
          n77 = xnode ("Register Write")("Data"=w406) -> ()  [unwired: 1 in, 1 out]
          n78 = And(x=w403, y=w402) -> (x .and. y?=w404:bool)
          "Z Reference Loop iterations" <- w405
        }
        n79 = while {
          tunnel: w129 -> [w416]
          shift-right: [w414] -> _
          shift-left: FALSE ("Data") -> [w413]
          i -> [w417]
          stop <- w415 stop-if-true
          n80 = node-c288() -> (w429:T15)  [unwired: 1 in]
          n81 = timed-loop {
            timing: w429 -> [_]
            timing-out: [_] -> w428
            tunnel: "DT Duty Cycle (periods)" -> [w440]
            tunnel: w416 -> [w439]
            tunnel: [w438] -> w424
            tunnel: "DT Reset" -> [w437]
            tunnel: "DT Phase Offset (periods)" -> [w435]
            stop <- TRUE stop-if-true
            n82 = call "Square Wave Generator2"("frequency (periods/tick)"=w439, "reset"=w437, "phase offset (periods)"=w435, "duty cycle (periods)"=w440) -> ("square wave out"=w438:bool)  [unwired: 11 in]
          }
          n83 = call "Loop Timer7"("Count(uSec)"="Trigger Generation Time Period (uSec)") -> ()  [unwired: 1 out]
          n84 = Add(x="DT Reference DC Offset (V)", y="DT Reference Amplitude (V)") -> (x+y=w421:fxp<+/-,32,16>)
          n85 = Subtract(x="DT Reference DC Offset (V)", y="DT Reference Amplitude (V)") -> (x-y=w420:fxp<+/-,32,16>)
          n86 = node-c288(w428) -> ()
          n87 = Select(t=w421, s=w424, f=w420) -> (s? t:f=w418:fxp<+/-,32,16>)
          n88 = xnode ("Register Write")("Data"=w424) -> ()  [unwired: 1 in, 1 out]
          n89 = call "measure_loop_rate_FPGA.vi"() -> ("Loop Rate (Ticks)"=→"Measured Trigger Generation Loop Period (Ticks)":u32)  [unwired: 11 in]
          n90 = xnode ("Register Read")() -> ("Data"=w414:bool)  [unwired: 1 in, 1 out]
          n91 = In Range and Coerce(upper limit="Detector Trigger Upper Limit (V)", x=w418, lower limit="Detector Trigger Lower Limit (V)") -> (coerced(x)=w419:fxp<+/-,32,16>, In Range?=→"Detector Trigger In Range?":bool)
          n92 = xnode ("Register Write")("Data"=w419) -> ()  [unwired: 1 in, 1 out]
          n93 = And(x=w414, y=w413) -> (x .and. y?=w415:bool)
          "Trigger Generation Loop iterations" <- w417
        }
        n94 = while {
          tunnel: [w454] -> w136
          shift-right: [w446] -> _
          shift-left: FALSE ("Data") -> [w445]
          i -> [w448]
          stop <- w456 stop-if-true
          n95 = xnode ("Register Read")() -> ("Data"=w449:fxp<+/-,32,16>)  [unwired: 1 in, 1 out]
          n96 = xnode ("Register Read")() -> ("Data"=w452:fxp<+/-,24,5>)  [unwired: 1 in, 1 out]
          n97 = xnode ("Register Read")() -> ("Data"=w451:fxp<+/-,24,5>)  [unwired: 1 in, 1 out]
          n98 = xnode ("Register Read")() -> ("Data"=w450:fxp<+/-,24,5>)  [unwired: 1 in, 1 out]
          n99 = xnode "FPGA I/O Node"("Mod8/AO0"=w452, "Mod8/AO1"=w451, "Mod8/AO2"=w450, "Mod8/AO3"=w449) -> ("error out"=w454:errorcluster)  [unwired: 5 in, 4 out]
          n100 = call "Loop Timer4"("Count(uSec)"="Module Output Loop Period (uSec)") -> ()  [unwired: 1 out]
          n101 = xnode ("Register Read")() -> ("Data"=w446:bool)  [unwired: 1 in, 1 out]
          n102 = call "measure_loop_rate_FPGA.vi"() -> ("Loop Rate (Ticks)"=→"Measured Module Output Loop Period (Ticks)":u32)  [unwired: 11 in]
          n103 = Unbundle By Name(w454) -> ("status"=w455:bool)
          n104 = And(x=w446, y=w445) -> (x .and. y?=w447:bool)
          n105 = Or(x=w455, y=w447) -> (x .or. y?=w456:bool)
          "Module output loop iterations" <- w448
        }
        n106 = Equal?(x="Data Save Trigger Source", y=Data_Save_Trigger."Detector") -> (x = y?=w131:bool)
        n107 = case shown="\"Fly\", Default" w130 {
          tunnel: [w142 errorcluster {"Status?"=FALSE, "Code"=0, "Source"=""} ("error out")] -> w139
          tunnel: "Data Save Flag" -> [w141 _]
          tunnel: w131 -> [w140 _]
          frame "Fly", Default {
            n108 = case shown="\"Save Data\"" w141 {
              tunnel: [errorcluster {"Status?"=FALSE, "Code"=0, "Source"=""} ("error out") w147] -> w142
              tunnel: w140 -> [_ w146]
              frame "Skip Data", Default {
              }
              frame "Save Data" {
                n109 = while {
                  tunnel: [w150] -> w147
                  shift-right: [w160] -> _
                  shift-left: FALSE ("Data") -> [w161]
                  tunnel: w146 -> [w154]
                  shift-right: [w153] -> _
                  shift-left: FALSE ("Data") -> [w151]
                  i -> [w158]
                  stop <- w163 stop-if-true
                  n110 = Not(x=w161) -> (.not. x?=w159:bool)
                  n111 = xnode ("Register Read")() -> ("Data"=w160:bool)  [unwired: 1 in, 1 out]
                  n112 = call "Loop Timer2"("Count(uSec)"="FIFO Loop Period (us)") -> ()  [unwired: 1 out]
                  n113 = And(x=w160, y=w159) -> (x .and. y?=w156:bool)
                  n114 = Select(t=w156, s=w154, f=TRUE) -> (s? t:f=w157:bool)
                  n115 = case shown="True" w157 {
                    tunnel: [errorcluster {"Status?"=FALSE, "Code"=0, "Source"=""} ("error out") w174] -> w150
                    tunnel: [FALSE ("Status?") w173] -> w149
                    tunnel: [FALSE w172] -> w148
                    frame False {
                    }
                    frame True {
                      w191 = 5  # # of Data Strings
                      n116 = local read "Measured Controller Loop Period (Ticks)"() -> (w169:u32)
                      n117 = xnode ("Register Read")() -> ("Data"=w186:fxp<+/-,32,16>)  [unwired: 1 in, 1 out]
                      n118 = xnode ("Register Read")() -> ("Data"=w187:fxp<+/-,32,16>)  [unwired: 1 in, 1 out]
                      n119 = xnode ("Register Read")() -> ("Data"=w188:fxp<+/-,32,16>)  [unwired: 1 in, 1 out]
                      n120 = xnode ("Register Read")() -> ("Data"=w177:fxp<+/-,24,5>)  [unwired: 1 in, 1 out]
                      n121 = xnode ("Register Read")() -> ("Data"=w178:fxp<+/-,24,5>)  [unwired: 1 in, 1 out]
                      n122 = xnode ("Register Read")() -> ("Data"=w179:fxp<+/-,24,5>)  [unwired: 1 in, 1 out]
                      n123 = xnode ("Register Read")() -> ("Data"=w180:fxp<+/-,32,16>)  [unwired: 1 in, 1 out]
                      n124 = xnode ("Register Read")() -> ("Data"=w181:fxp<+/-,32,16>)  [unwired: 1 in, 1 out]
                      n125 = xnode ("Register Read")() -> ("Data"=w182:fxp<+/-,32,16>)  [unwired: 1 in, 1 out]
                      n126 = xnode ("Register Read")() -> ("Data"=w183:fxp<+/-,32,16>)  [unwired: 1 in, 1 out]
                      n127 = xnode ("Register Read")() -> ("Data"=w184:fxp<+/-,32,16>)  [unwired: 1 in, 1 out]
                      n128 = xnode ("Register Read")() -> ("Data"=w185:fxp<+/-,32,16>)  [unwired: 1 in, 1 out]
                      n129 = xnode ("Register Read")() -> ("Data"=w189:fxp<+/-,32,16>)  [unwired: 1 in, 1 out]
                      n130 = local read "Measured XY Reference Loop Period (ticks)"() -> (w168:u32)
                      n131 = case shown="\"Data Log 2\"" "Datalog Cases" {
                        tunnel: fxp<+/-,58,25> 0.0 ("fixed-point type") -> [w209 w223 w231 w243 w253 w268 w281 w292 w310 w322 w332 w344 w356 w366 w376 w389]
                        tunnel: [w217 w228 w240 w251 w264 w277 w288 w304 w314 w328 w337 w352 w363 w373 w383 w395] -> w196
                        tunnel: w186 -> [w208 _ _ _ w252 _ _ _ _ _ _ _ _ _ _ w386]
                        tunnel: w177 -> [w214 _ _ _ w257 _ _ _ _ w329 _ _ w359 _ _ _]
                        tunnel: w178 -> [_ w227 _ _ _ w272 _ _ _ _ w342 _ _ w369 _ _]
                        tunnel: w179 -> [_ _ w237 _ _ _ w285 _ _ _ _ w353 _ _ w379 _]
                        tunnel: [w216 w222 w239 w245 w263 w276 w287 w300 w313 w323 w336 w351 w362 w372 w382 w394] -> w195
                        tunnel: [w215 w229 w238 w250 w262 w275 w286 w296 w312 w324 w335 w350 w361 w371 w381 w393] -> w194
                        tunnel: w180 -> [w211 _ _ w247 w259 _ _ w307 _ w327 w341 w348 w358 _ _ w391]
                        tunnel: w181 -> [_ w224 _ w246 _ w271 _ w303 _ w326 w340 w347 _ w368 _ w390]
                        tunnel: fxp<+/-,40,17> 0.0 ("fixed-point type") -> [_ _ w233 w241 w255 w267 w279 w291 w308 w319 w331 w343 w355 w365 w375 _]
                        tunnel: w182 -> [_ _ w234 w244 _ _ w284 w299 _ w320 w339 w346 _ _ w378 _]
                        tunnel: w183 -> [_ _ _ _ w258 _ _ w306 w317 _ _ _ _ _ _ _]
                        tunnel: w184 -> [_ _ _ _ _ w270 _ w302 w316 _ _ _ _ _ _ _]
                        tunnel: w185 -> [_ _ _ _ _ _ w283 w298 w315 _ _ _ _ _ _ _]
                        tunnel: w187 -> [_ w220 _ _ _ w265 _ _ _ _ _ _ _ _ _ w385]
                        tunnel: w188 -> [_ _ w230 _ _ _ w278 _ _ _ _ _ _ _ _ _]
                        tunnel: [w213 w226 w236 w249 w261 w274 w282 w295 w311 w325 w334 w349 w360 w370 w380 w392] -> w192
                        tunnel: w191 -> [w212 w225 w235 w248 w260 w273 w289 w294 w318 w330 w338 w354 w364 w374 w384 w396]
                        tunnel: [w212 w225 w235 w248 w260 w273 w289 w294 w318 w330 w338 w354 w364 w374 w384 w396] -> w176
                        tunnel: w189 -> [_ _ _ _ _ _ _ _ _ _ _ _ _ _ _ w388]
                        tunnel: [w210 w221 w232 w242 w254 w266 w280 w293 w309 w321 w333 w345 w357 w367 w377 w387] -> w190
                        tunnel: w169 -> [w207 w219 _ _ _ _ _ _ _ _ _ _ _ _ _ _]
                        tunnel: w168 -> [w206 w218 _ _ _ _ _ _ _ _ _ _ _ _ _ _]
                        frame "Data Log 1", Default {
                          n132 = To Fixed-Point(fixed-point type=w209, number=w208) -> (fixed-point=w217:fxp<+/-,58,25>)
                          n133 = To Fixed-Point(fixed-point type=w209, number=w214) -> (fixed-point=w216:fxp<+/-,58,25>)
                          n134 = To Fixed-Point(fixed-point type=w209, number=w211) -> (fixed-point=w215:fxp<+/-,58,25>)
                          n135 = To Fixed-Point(fixed-point type=w209, number=w207) -> (fixed-point=w213:fxp<+/-,58,25>)
                          n136 = To Fixed-Point(fixed-point type=w209, number=w206) -> (fixed-point=w210:fxp<+/-,58,25>)
                        }
                        frame "Data Log 2" {
                          n137 = To Fixed-Point(fixed-point type=w223, number=w220) -> (fixed-point=w228:fxp<+/-,58,25>)
                          n138 = To Fixed-Point(fixed-point type=w223, number=w227) -> (fixed-point=w222:fxp<+/-,58,25>)
                          n139 = To Fixed-Point(fixed-point type=w223, number=w224) -> (fixed-point=w229:fxp<+/-,58,25>)
                          n140 = To Fixed-Point(fixed-point type=w223, number=w219) -> (fixed-point=w226:fxp<+/-,58,25>)
                          n141 = To Fixed-Point(fixed-point type=w223, number=w218) -> (fixed-point=w221:fxp<+/-,58,25>)
                        }
                        frame "Data Log 3" {
                          n142 = To Fixed-Point(fixed-point type=w231, number=w230) -> (fixed-point=w240:fxp<+/-,58,25>)
                          n143 = To Fixed-Point(fixed-point type=w231, number=w237) -> (fixed-point=w239:fxp<+/-,58,25>)
                          n144 = To Fixed-Point(fixed-point type=w231, number=w234) -> (fixed-point=w238:fxp<+/-,58,25>)
                          n145 = To Fixed-Point(fixed-point type=w231, number=w233) -> (fixed-point=w236:fxp<+/-,58,25>)
                          n146 = To Fixed-Point(fixed-point type=w231, number=w233) -> (fixed-point=w232:fxp<+/-,58,25>)
                        }
                        frame "Data Log 4" {
                          n147 = To Fixed-Point(fixed-point type=w243, number=w247) -> (fixed-point=w251:fxp<+/-,58,25>)
                          n148 = To Fixed-Point(fixed-point type=w243, number=w246) -> (fixed-point=w245:fxp<+/-,58,25>)
                          n149 = To Fixed-Point(fixed-point type=w243, number=w244) -> (fixed-point=w250:fxp<+/-,58,25>)
                          n150 = To Fixed-Point(fixed-point type=w243, number=w241) -> (fixed-point=w249:fxp<+/-,58,25>)
                          n151 = To Fixed-Point(fixed-point type=w243, number=w241) -> (fixed-point=w242:fxp<+/-,58,25>)
                        }
                        frame "Data Log 5" {
                          n152 = To Fixed-Point(fixed-point type=w253, number=w252) -> (fixed-point=w264:fxp<+/-,58,25>)
                          n153 = Subtract(x=w259, y=w258) -> (x-y=w256:fxp<+/-,33,17>)
                          n154 = To Fixed-Point(fixed-point type=w253, number=w257) -> (fixed-point=w263:fxp<+/-,58,25>)
                          n155 = To Fixed-Point(fixed-point type=w253, number=w256) -> (fixed-point=w262:fxp<+/-,58,25>)
                          n156 = To Fixed-Point(fixed-point type=w253, number=w255) -> (fixed-point=w261:fxp<+/-,58,25>)
                          n157 = To Fixed-Point(fixed-point type=w253, number=w255) -> (fixed-point=w254:fxp<+/-,58,25>)
                        }
                        frame "Data Log 6" {
                          n158 = To Fixed-Point(fixed-point type=w268, number=w265) -> (fixed-point=w277:fxp<+/-,58,25>)
                          n159 = To Fixed-Point(fixed-point type=w268, number=w272) -> (fixed-point=w276:fxp<+/-,58,25>)
                          n160 = Subtract(x=w271, y=w270) -> (x-y=w269:fxp<+/-,33,17>)
                          n161 = To Fixed-Point(fixed-point type=w268, number=w269) -> (fixed-point=w275:fxp<+/-,58,25>)
                          n162 = To Fixed-Point(fixed-point type=w268, number=w267) -> (fixed-point=w274:fxp<+/-,58,25>)
                          n163 = To Fixed-Point(fixed-point type=w268, number=w267) -> (fixed-point=w266:fxp<+/-,58,25>)
                        }
                        frame "Data Log 7" {
                          n164 = To Fixed-Point(fixed-point type=w281, number=w278) -> (fixed-point=w288:fxp<+/-,58,25>)
                          n165 = To Fixed-Point(fixed-point type=w281, number=w285) -> (fixed-point=w287:fxp<+/-,58,25>)
                          n166 = Subtract(x=w284, y=w283) -> (x-y=w290:fxp<+/-,33,17>)
                          n167 = To Fixed-Point(fixed-point type=w281, number=w290) -> (fixed-point=w286:fxp<+/-,58,25>)
                          n168 = To Fixed-Point(fixed-point type=w281, number=w279) -> (fixed-point=w282:fxp<+/-,58,25>)
                          n169 = To Fixed-Point(fixed-point type=w281, number=w279) -> (fixed-point=w280:fxp<+/-,58,25>)
                        }
                        frame "Data Log 8" {
                          n170 = Subtract(x=w307, y=w306) -> (x-y=w305:fxp<+/-,33,17>)
                          n171 = Subtract(x=w303, y=w302) -> (x-y=w301:fxp<+/-,33,17>)
                          n172 = To Fixed-Point(fixed-point type=w292, number=w305) -> (fixed-point=w304:fxp<+/-,58,25>)
                          n173 = Subtract(x=w299, y=w298) -> (x-y=w297:fxp<+/-,33,17>)
                          n174 = To Fixed-Point(fixed-point type=w292, number=w301) -> (fixed-point=w300:fxp<+/-,58,25>)
                          n175 = To Fixed-Point(fixed-point type=w292, number=w297) -> (fixed-point=w296:fxp<+/-,58,25>)
                          n176 = To Fixed-Point(fixed-point type=w292, number=w291) -> (fixed-point=w295:fxp<+/-,58,25>)
                          n177 = To Fixed-Point(fixed-point type=w292, number=w291) -> (fixed-point=w293:fxp<+/-,58,25>)
                        }
                        frame "Data Log 9" {
                          n178 = To Fixed-Point(fixed-point type=w310, number=w317) -> (fixed-point=w314:fxp<+/-,58,25>)
                          n179 = To Fixed-Point(fixed-point type=w310, number=w316) -> (fixed-point=w313:fxp<+/-,58,25>)
                          n180 = To Fixed-Point(fixed-point type=w310, number=w315) -> (fixed-point=w312:fxp<+/-,58,25>)
                          n181 = To Fixed-Point(fixed-point type=w310, number=w308) -> (fixed-point=w311:fxp<+/-,58,25>)
                          n182 = To Fixed-Point(fixed-point type=w310, number=w308) -> (fixed-point=w309:fxp<+/-,58,25>)
                        }
                        frame "Data Log 10" {
                          n183 = To Fixed-Point(fixed-point type=w322, number=w329) -> (fixed-point=w328:fxp<+/-,58,25>)
                          n184 = To Fixed-Point(fixed-point type=w322, number=w327) -> (fixed-point=w323:fxp<+/-,58,25>)
                          n185 = To Fixed-Point(fixed-point type=w322, number=w326) -> (fixed-point=w324:fxp<+/-,58,25>)
                          n186 = To Fixed-Point(fixed-point type=w322, number=w320) -> (fixed-point=w325:fxp<+/-,58,25>)
                          n187 = To Fixed-Point(fixed-point type=w322, number=w319) -> (fixed-point=w321:fxp<+/-,58,25>)
                        }
                        frame "Data Log 11" {
                          n188 = To Fixed-Point(fixed-point type=w332, number=w342) -> (fixed-point=w337:fxp<+/-,58,25>)
                          n189 = To Fixed-Point(fixed-point type=w332, number=w341) -> (fixed-point=w336:fxp<+/-,58,25>)
                          n190 = To Fixed-Point(fixed-point type=w332, number=w340) -> (fixed-point=w335:fxp<+/-,58,25>)
                          n191 = To Fixed-Point(fixed-point type=w332, number=w339) -> (fixed-point=w334:fxp<+/-,58,25>)
                          n192 = To Fixed-Point(fixed-point type=w332, number=w331) -> (fixed-point=w333:fxp<+/-,58,25>)
                        }
                        frame "Data Log 12" {
                          n193 = To Fixed-Point(fixed-point type=w344, number=w353) -> (fixed-point=w352:fxp<+/-,58,25>)
                          n194 = To Fixed-Point(fixed-point type=w344, number=w348) -> (fixed-point=w351:fxp<+/-,58,25>)
                          n195 = To Fixed-Point(fixed-point type=w344, number=w347) -> (fixed-point=w350:fxp<+/-,58,25>)
                          n196 = To Fixed-Point(fixed-point type=w344, number=w346) -> (fixed-point=w349:fxp<+/-,58,25>)
                          n197 = To Fixed-Point(fixed-point type=w344, number=w343) -> (fixed-point=w345:fxp<+/-,58,25>)
                        }
                        frame "Data Log 13" {
                          n198 = To Fixed-Point(fixed-point type=w356, number=w355) -> (fixed-point=w363:fxp<+/-,58,25>)
                          n199 = To Fixed-Point(fixed-point type=w356, number=w359) -> (fixed-point=w362:fxp<+/-,58,25>)
                          n200 = To Fixed-Point(fixed-point type=w356, number=w358) -> (fixed-point=w361:fxp<+/-,58,25>)
                          n201 = To Fixed-Point(fixed-point type=w356, number=w355) -> (fixed-point=w360:fxp<+/-,58,25>)
                          n202 = To Fixed-Point(fixed-point type=w356, number=w355) -> (fixed-point=w357:fxp<+/-,58,25>)
                        }
                        frame "Data Log 14" {
                          n203 = To Fixed-Point(fixed-point type=w366, number=w365) -> (fixed-point=w373:fxp<+/-,58,25>)
                          n204 = To Fixed-Point(fixed-point type=w366, number=w369) -> (fixed-point=w372:fxp<+/-,58,25>)
                          n205 = To Fixed-Point(fixed-point type=w366, number=w368) -> (fixed-point=w371:fxp<+/-,58,25>)
                          n206 = To Fixed-Point(fixed-point type=w366, number=w365) -> (fixed-point=w370:fxp<+/-,58,25>)
                          n207 = To Fixed-Point(fixed-point type=w366, number=w365) -> (fixed-point=w367:fxp<+/-,58,25>)
                        }
                        frame "Data Log 15" {
                          n208 = To Fixed-Point(fixed-point type=w376, number=w375) -> (fixed-point=w383:fxp<+/-,58,25>)
                          n209 = To Fixed-Point(fixed-point type=w376, number=w379) -> (fixed-point=w382:fxp<+/-,58,25>)
                          n210 = To Fixed-Point(fixed-point type=w376, number=w378) -> (fixed-point=w381:fxp<+/-,58,25>)
                          n211 = To Fixed-Point(fixed-point type=w376, number=w375) -> (fixed-point=w380:fxp<+/-,58,25>)
                          n212 = To Fixed-Point(fixed-point type=w376, number=w375) -> (fixed-point=w377:fxp<+/-,58,25>)
                        }
                        frame "Data Log 16" {
                          n213 = To Fixed-Point(fixed-point type=w389, number=w386) -> (fixed-point=w395:fxp<+/-,58,25>)
                          n214 = To Fixed-Point(fixed-point type=w389, number=w385) -> (fixed-point=w394:fxp<+/-,58,25>)
                          n215 = To Fixed-Point(fixed-point type=w389, number=w391) -> (fixed-point=w393:fxp<+/-,58,25>)
                          n216 = To Fixed-Point(fixed-point type=w389, number=w390) -> (fixed-point=w392:fxp<+/-,58,25>)
                          n217 = To Fixed-Point(fixed-point type=w389, number=w388) -> (fixed-point=w387:fxp<+/-,58,25>)
                        }
                      }
                      "Number of Data Strings" <- w176
                      n218 = Build Array(w196, w195, w194, w192, w190) -> (w175:fxp<+/-,58,25>[])
                      n219 = for {
                        N: w176 -> [_]
                        tunnel: w175 -> [w205] mode=indexing
                        shift-right: [w203] -> w174
                        shift-left: errorcluster {"Status?"=FALSE, "Code"=0, "Source"=""} ("error out") -> [w202]
                        shift-right: [w199] -> w172
                        shift-left: FALSE -> [w200]
                        n220 = xnode ("FIFO")("Element"=w205, "Timeout"="Timeout FPGA FIFO1", "error in (no error)"=w202) -> ("Timed Out?"=w201:bool, "error out"=w203:errorcluster)  [unwired: 1 in, 1 out]
                        "FIFO Timed Out?" <- w201
                        n221 = Or(x=w201, y=w200) -> (x .or. y?=w199:bool)
                      }
                      "FIFO Timed Out" <- w172
                      n222 = Unbundle By Name(w174) -> ("Status?"=w173:bool)
                    }
                  }
                  n223 = xnode ("Register Read")() -> ("Data"=w153:bool)  [unwired: 1 in, 1 out]
                  n224 = call "measure_loop_rate_FPGA.vi"() -> ("Loop Rate (Ticks)"=→"Measured Datalog Period (Ticks)":u32)  [unwired: 11 in]
                  n225 = And(x=w151, y=w153) -> (x .and. y?=w152:bool)
                  n226 = Compound Arithmetic op=OR(w149, w148, w152) -> (w163:bool)
                  n227 = case shown="True" w163 {
                    selector: w163 -> [_ w397]
                    frame False {
                    }
                    frame True {
                      n228 = xnode ("Register Write")("Data"=w397) -> ()  [unwired: 1 in, 1 out]
                      n229 = local write "Stop Scan"(w397) -> ()
                    }
                  }
                  "FIFO loop iterations" <- w158
                }
              }
            }
          }
          frame "Step" {
          }
        }
        n230 = Merge Errors(w136, w139) -> (w137:errorcluster)
        "Run Loop error" <- w137
        n231 = case shown="Error" w137 {
          tunnel: [FPGA_states."End Run" FPGA_states."Wait"] -> w138
          frame No Error {
          }
          frame Error {
            n232 = local write "Stop Scan"(TRUE) -> ()
          }
        }
      }
      frame "End Run" {
        n233 = flat-sequence {
          tunnel: w585 -> [w588]
          tunnel: [w588] -> w584
          frame #0 {
            n234 = xnode ("Register Write")("Data"=FALSE) -> ()  [unwired: 1 in, 1 out]
          }
        }
        "End Run Error" <- w585
      }
      frame "Shutdown" {
        n235 = xnode "FPGA I/O Node"("error in"=w592, "System Reset"=TRUE) -> ("error out"=w591:errorcluster)  [unwired: 1 in, 1 out]
        "Shutdown error" <- w591
      }
    }
    "FPGA state" <- w21
    "Outer Loop iterations" <- w13
  }
  n236 = while {
    tunnel: w1 -> [w608]
    shift-right: [w606] -> _
    shift-left: _ -> [w605]
    shift-right: [w603] -> _
    shift-left: u8 0 ("USER FPGA LED") -> [w601]
    stop <- FALSE stop-if-true
    # "Heartbeat Loop - monitors errors and relays status to RT and LED on cRIO"
    n237 = local read "Interferometer Loop Error"() -> (w595:errorcluster)
    n238 = local read "Shutdown error"() -> (w610:errorcluster)
    n239 = local read "Run Loop error"() -> (w613:errorcluster)
    n240 = local read "Start Run Error"() -> (w612:errorcluster)
    n241 = local read "End Run Error"() -> (w609:errorcluster)
    n242 = local read "Wait error"() -> (w611:errorcluster)
    n243 = Merge Errors(w605, w613, w612, w611, w610, w609, w595, w608) -> (w607:errorcluster)
    "FPGA error monitor" <- w607
    n244 = Unbundle By Name(w607) -> ("status"=w596:bool)
    n245 = Not Equal?(x=w601, y=u8 0) -> (x != y?=w599:bool)
    n246 = case shown="False" w596 {
      tunnel: [u16 500 ("Count(mSec)") u16 100 ("Count(mSec)")] -> w604
      tunnel: [u8 1 ("USER FPGA LED") u8 2 ("USER FPGA LED")] -> w597
      frame False {
        # "Set LED green \nand rep rate to 1 Hz"
      }
      frame True {
        # "Set LED yellow \nand rep rate to 5 Hz"
      }
    }
    n247 = Select(t=u8 0, s=w599, f=w597) -> (s? t:f=w603:u8)
    n248 = xnode "FPGA I/O Node"("USER FPGA LED"=w603) -> ("error out"=w606:errorcluster)  [unwired: 2 in, 1 out]
    n249 = call "Loop Timer12"("Count(mSec)"=w604) -> ()  [unwired: 1 out]
  }
  n250 = while {
    i -> [w618]
    stop <- FALSE stop-if-true
    n251 = xnode ("Register Read")() -> ("Data"=w622:i32)  [unwired: 1 in, 1 out]
    n252 = xnode ("Register Read")() -> ("Data"=w623:i32)  [unwired: 1 in, 1 out]
    n253 = xnode ("Register Read")() -> ("Data"=w624:i32)  [unwired: 1 in, 1 out]
    n254 = xnode ("Register Read")() -> ("Data"=w619:i32)  [unwired: 1 in, 1 out]
    n255 = xnode ("Register Read")() -> ("Data"=w620:i32)  [unwired: 1 in, 1 out]
    n256 = xnode ("Register Read")() -> ("Data"=w621:i32)  [unwired: 1 in, 1 out]
    n257 = call "Loop Timer5"("Count(uSec)"="Plant Output Loop Period (uSec)") -> ()  [unwired: 1 out]
    n258 = call "measure_loop_rate_FPGA.vi"() -> ("Loop Rate (Ticks)"=→"Measured Plant Output Loop Period (Ticks)":u32)  [unwired: 11 in]
    n259 = Multiply(x=w619, y="Optics X Stage Resolution (nm)") -> (x*y=w637:fxp<+/-,32,16>)
    "Optics X Stage Displacement raw (nm)" <- w637
    n260 = Multiply(x=w622, y="Sample X Stage Resolution (nm)") -> (x*y=w631:fxp<+/-,32,16>)
    "Sample X Stage Displacement raw (nm)" <- w631
    n261 = Multiply(x=w620, y="Optics Y Stage Resolution (nm)") -> (x*y=w634:fxp<+/-,32,16>)
    "Optics Y Stage Displacement raw (nm)" <- w634
    n262 = Multiply(x=w623, y="Sample Y Stage Resolution (nm)") -> (x*y=w630:fxp<+/-,32,16>)
    "Sample Y Stage Displacement raw (nm)" <- w630
    n263 = Multiply(x=w621, y="Optics Z Stage Resolution (nm)") -> (x*y=w632:fxp<+/-,32,16>)
    "Optics Z Stage Displacement raw (nm)" <- w632
    n264 = Multiply(x=w624, y="Sample Z Stage Resolution (nm)") -> (x*y=w629:fxp<+/-,32,16>)
    "Sample Z Stage Displacement raw (nm)" <- w629
    n265 = xnode ("Register Write")("Data"=w637) -> ()  [unwired: 1 in, 1 out]
    n266 = xnode ("Register Write")("Data"=w634) -> ()  [unwired: 1 in, 1 out]
    n267 = xnode ("Register Write")("Data"=w632) -> ()  [unwired: 1 in, 1 out]
    n268 = xnode ("Register Write")("Data"=w631) -> ()  [unwired: 1 in, 1 out]
    n269 = xnode ("Register Write")("Data"=w630) -> ()  [unwired: 1 in, 1 out]
    n270 = xnode ("Register Write")("Data"=w629) -> ()  [unwired: 1 in, 1 out]
    "Plant output loop iterations" <- w618
  }
  n271 = node-c288(refnum<k21> "40 MHz Onboard Clock" ("Source Name"), w1) -> (w6:T15)
  n272 = timed-loop {
    timing: w6 -> [_]
    timing-out: [_] -> w5
    shift-right: [w678] -> _
    shift-left: _ -> [w680]
    shift-right: [w677] -> _
    shift-left: _ -> [w679]
    shift-right: [w644] -> _
    shift-left: w4 -> [w691]
    shift-right: [w693] -> _
    shift-left: u32 0 ("Tick Count(Ticks)") -> [w692]
    shift-right: [w669] -> _
    shift-left: _ -> [w668]
    shift-right: [w670] -> _
    shift-left: _ -> [w667]
    shift-right: [w646] -> _
    shift-left: w4 -> [w688]
    shift-right: [w657] -> _
    shift-left: _ -> [w658]
    shift-right: [w656] -> _
    shift-left: _ -> [w659]
    shift-right: [w642] -> _
    shift-left: w4 -> [w684]
    shift-right: [w675] -> _
    shift-left: _ -> [w673]
    shift-right: [w674] -> _
    shift-left: _ -> [w672]
    shift-right: [w645] -> _
    shift-left: w4 -> [w690]
    shift-right: [w662] -> _
    shift-left: _ -> [w663]
    shift-right: [w661] -> _
    shift-left: _ -> [w664]
    shift-right: [w643] -> _
    shift-left: w4 -> [w686]
    shift-right: [w652] -> _
    shift-left: _ -> [w654]
    shift-right: [w653] -> _
    shift-left: _ -> [w655]
    shift-right: [w641] -> _
    shift-left: w4 -> [w682]
    shift-right: [w649] -> _
    shift-left: _ -> [w648]
    i -> [w640]
    stop <- w647 stop-if-true
    # "Tracks interferometer data"
    n273 = xnode "FPGA I/O Node"("error in"=w648) -> ("error out"=w671:errorcluster, "Mod4/DIO2"=w675:bool, "Mod4/DIO3"=w674:bool)  [unwired: 2 in, 2 out]
    "Mod4/DIO2" <- w675
    "Mod4/DIO3" <- w674
    n274 = xnode "FPGA I/O Node"("error in"=w648) -> ("error out"=w665:errorcluster, "Mod5/DIO2"=w662:bool, "Mod5/DIO3"=w661:bool)  [unwired: 2 in, 2 out]
    "Mod5/DIO2" <- w662
    "Mod5/DIO3" <- w661
    n275 = xnode "FPGA I/O Node"("error in"=w648) -> ("error out"=w651:errorcluster, "Mod6/DIO0"=w657:bool, "Mod6/DIO1"=w656:bool)  [unwired: 2 in, 2 out]
    "Mod6/DIO0" <- w657
    "Mod6/DIO1" <- w656
    n276 = xnode "FPGA I/O Node"("error in"=w648) -> ("error out"=w666:errorcluster, "Mod5/DIO0"=w669:bool, "Mod5/DIO1"=w670:bool)  [unwired: 2 in, 2 out]
    "Mod5/DIO0" <- w669
    "Mod5/DIO1" <- w670
    n277 = xnode ("FPGA I/O Node")("error in"=w648) -> ("error out"=w676:errorcluster, "Mod4/DIO0"=w678:bool, "Mod4/DIO1"=w677:bool)  [unwired: 2 in, 2 out]
    "Mod4/DIO0" <- w678
    "Mod4/DIO1" <- w677
    n278 = xnode "FPGA I/O Node"("error in"=w648) -> ("error out"=w650:errorcluster, "Mod6/DIO2"=w652:bool, "Mod6/DIO3"=w653:bool)  [unwired: 2 in, 2 out]
    "Mod6/DIO2" <- w652
    "Mod6/DIO3" <- w653
    n279 = call "Tick Count"() -> ("Tick Count(Ticks)"=w693:u32)
    n280 = Subtract(x=w693, y=w692) -> (x-y=→"Measured Counter Time Period (Ticks)":u32)
    n281 = Merge Errors(w676, w671, w666, w665, w651, w650) -> (w649:errorcluster)
    "Interferometer Loop Error" <- w649
    n282 = call "Quadrature.vi"("Reset Counter"="Reset Optics X", "Quad A"=w678, "ticks in"=w691, "Last Quad B"=w679, "Last Quad A"=w680, "Quad B"=w677) -> ("ticks out"=w644:i32)  [unwired: 5 in]
    n283 = call "Quadrature.vi"("Reset Counter"="Reset Sample X", "Quad A"=w675, "ticks in"=w690, "Last Quad B"=w672, "Last Quad A"=w673, "Quad B"=w674) -> ("ticks out"=w645:i32)  [unwired: 5 in]
    n284 = call "Quadrature.vi"("Reset Counter"="Reset Optics Y", "Quad A"=w669, "ticks in"=w688, "Last Quad B"=w667, "Last Quad A"=w668, "Quad B"=w670) -> ("ticks out"=w646:i32)  [unwired: 5 in]
    n285 = call "Quadrature.vi"("Reset Counter"="Reset Sample Y", "Quad A"=w662, "ticks in"=w686, "Last Quad B"=w664, "Last Quad A"=w663, "Quad B"=w661) -> ("ticks out"=w643:i32)  [unwired: 5 in]
    n286 = call "Quadrature.vi"("Reset Counter"="Reset Optics Z", "Quad A"=w657, "ticks in"=w684, "Last Quad B"=w659, "Last Quad A"=w658, "Quad B"=w656) -> ("ticks out"=w642:i32)  [unwired: 5 in]
    n287 = call "Quadrature.vi"("Reset Counter"="Reset Sample Z", "Quad A"=w652, "ticks in"=w682, "Last Quad B"=w655, "Last Quad A"=w654, "Quad B"=w653) -> ("ticks out"=w641:i32)  [unwired: 5 in]
    n288 = xnode ("Register Write")("Data"=w646) -> ()  [unwired: 1 in, 1 out]
    n289 = xnode ("Register Write")("Data"=w644) -> ()  [unwired: 1 in, 1 out]
    n290 = xnode ("Register Write")("Data"=w645) -> ()  [unwired: 1 in, 1 out]
    n291 = xnode ("Register Write")("Data"=w643) -> ()  [unwired: 1 in, 1 out]
    n292 = Unbundle By Name(w649) -> ("status"=w647:bool)
    n293 = xnode ("Register Write")("Data"=w642) -> ()  [unwired: 1 in, 1 out]
    n294 = xnode ("Register Write")("Data"=w641) -> ()  [unwired: 1 in, 1 out]
    "Counter Loop iterations" <- w640
  }
  n295 = node-c288(w5) -> ()  [unwired: 1 out]
